vi "ONR Det Tube.vi"() -> ()   [LabVIEW 2018]
uses:
  <vilib>/Utility/miscctls.llb/LVPointTypeDef.ctl
  <vilib>/DAQmx/write.llb/DAQmx Write (Digital 1D Bool 1Chan 1Samp).vi
  <vilib>/Analysis/baseanly.llb/Mean (DBL).vi
  <vilib>/DAQmx/read.llb/DAQmx Read (Analog 1D Wfm NChan 1Samp).vi
  <vilib>/DAQmx/create/channels.llb/DAQmx Create Channel (DO-Digital Output).vi
  <vilib>/DAQmx/miscellaneous.llb/DAQmx Fill In Error Info.vi
  <vilib>/Utility/file.llb/Write Delimited Spreadsheet (string).vi
  <vilib>/Analysis/NI_AALBase.lvlib
panel:
  in  "Stop sensors":bool
  in  "Stop all":bool
  out "log_manifold_vent_end":timestamp
  out "log_manifold_vent_start":timestamp
  out "log_end_time":timestamp
  out "log_start_time":timestamp
  in  "Sensor sample period (ms)":i32=100
  in  "Vacuum Cutoff":dbl[unit]=3447.37894475789 caption="Nominal" format="%.2f"
  out "vac err":dbl caption="Error" format="%.3f %%"
  out "Diluent Cutoff (default)":dbl[unit] caption="Nominal" format="%.2f"
  out "Fuel Cutoff (default)":dbl[unit] caption="Nominal" format="%.2f"
  out "dil err":dbl caption="Error" format="%.3f %%"
  in  "Diluent underpressure":dbl[unit]=160.0 caption="Undershoot" format="%.2f"
  out "diode read status":string="Diode read N/A"
  out "Pressure Unsafe?":bool
  in  "Atmospheric Pressure":dbl[unit] format="%.2f"
  out "Tube Pressure":dbl[unit] format="%.2f"
  out "Tube Temp":dbl[unit]=294.2611111111111 format="%.2f"
  out "Ambient Temp":dbl[unit]=294.2611111111111 format="%.2f"
  in  "Plot Units":string(combo)="Pa"
  out "System Pressures":waveform(dbl)[](graph)
  in  "Spark":bool
  out "Test row":string[](array[string])
  in  "Diluent":string(combo)
  in  "Equivalence Ratio":string(combo)
  in  "Diluent Mole Fraction":string(combo)
  in  "Fuel":string(combo)
  in  "Initial Pressure":string(combo)
  in  "Oxidizer":string(combo)
  out "Test CSV":string[][](array[string])
  out "Test CSV Header":string[](array[string])
  out "indices":T1
  in  "Run Test":bool
  in  "Test condition CSV":path=path "C:/DAQ/test matrix.csv" caption="Test Conditions"
  out "tube ready?":bool
  out "Test Status":string="No tests loaded"
  out "log_vac_press":dbl[](array[numeric])
  out "log_vac_time":timestamp[](array[timestamp])
  out "log_vac_temp":dbl[](array[numeric])
  out "valve\nrefs":refnum<vi>[](array[refnum])
  out "log_dil_press":dbl[](array[numeric])
  out "log_dil_time":timestamp[](array[timestamp])
  out "log_dil_temp":dbl[](array[numeric])
  out "is diluted?":bool
  out "Vacuum Cutoff (actual)":dbl[unit] caption="Measured" format="%.2f"
  out "f_a_st":dbl caption="F/Ast" format="%.6f"
  out "Oxidizer Cutoff (default)":dbl[unit] caption="Nominal" format="%.2f"
  out "ox err":dbl caption="Error" format="%.3f %%"
  out "Diluent Cutoff (actual)":dbl[unit] caption="Measured" format="%.2f"
  out "Oxidizer Cutoff (actual)":dbl[unit] caption="Measured" format="%.2f"
  out "phi actual":dbl caption="Equivalence" format="%_6g"
  out "dil_mf_measured":dbl caption="Dilution" format="%_6g"
  out "log_ox_press":dbl[](array[numeric])
  out "log_ox_time":timestamp[](array[timestamp])
  out "log_ox_temp":dbl[](array[numeric])
  out "Manifold Temp":dbl[unit]=294.2611111111111 format="%.2f"
  out "Diluent Cutoff (adjusted)":dbl[unit] caption="Adjusted" format="%.2f"
  out "Fuel Cutoff (actual)":dbl[unit] caption="Measured" format="%.2f"
  out "log_fuel_press":dbl[](array[numeric])
  out "log_fuel_time":timestamp[](array[timestamp])
  out "log_fuel_temp":dbl[](array[numeric])
  in  "Pressure measure time":dbl[unit]=30.0
  out "Fuel Cutoff (adjusted)":dbl[unit] caption="Adjusted" format="%.2f"
  out "Manifold Pressure":dbl[unit] format="%.2f"
  out "fuel err":dbl caption="Error" format="%.3f %%"
  in  "Fuel underpressure":dbl[unit]=180.0 caption="Undershoot" format="%.2f"
  in  "Mix Fan":bool
  in  "Valve Tube Inlet":bool caption="Tube Inlet"
  in  "Valve Mix Inlet":bool caption="Mix Inlet"
  in  "Valve Mix Outlet":bool caption="Mix Outlet"
  in  "Valve Tube Outlet":bool=TRUE caption="Tube Outlet"
  in  "Valve Oxidizer":bool caption="Oxidizer"
  in  "Valve Fuel":bool caption="Fuel"
  in  "Valve Diluent":bool caption="Diluent"
  in  "Valve Purge":bool caption="Purge"
  in  "Valve Vacuum":bool caption="Vacuum"
  in  "Set Mode":bool=TRUE
  out "Remaining":dbl format="%<%M:%S>t"
  in  "Stop":bool
  in  "Mix Time":dbl[unit]=180.0 format="%#_13g"
  in  "Mix Section Purge":dbl[unit]=30.0 format="%#_13g"
  in  "Tube Purge":dbl[unit]=360.0 format="%#_13g"
  in  "Tube State":T2(ring)
  # "Timing"
  # "Vacuum"
  # "Diluent"
  # "Oxidizer"
  # "Fuel"
types:
  T1 = cluster{"fuel":i32, "oxidizer":i32, "diluent":i32, "diluent_mol_frac":i32, "equivalence":i32, "init_pressure":i32, "p_f":i32, "p_ox":i32, "p_dil":i32}
  T2 = enum16{"Tube Vent", "Mix Section Purge", "Tube Purge", "Tube Vacuum", "Diluent Fill", "Oxidizer Fill", "Fuel Fill", "Fill Hold", "Mixing", "Tube Closed", "Ignition", "Manifold Vent"}
  T3 = enum8{"Enabled", "Disabled", "Disabled and Grayed Out"}
  T4 = typedef "LVPointTypeDef.ctl" = cluster{"Horizontal":i16, "Vertical":i16}
  T5 = typedef "LVRangeTypeDef.ctl" = cluster{"Minimum":dbl, "Maximum":dbl, "Increment":dbl, "Minor Increment":dbl, "Start":dbl}
  T6 = enum16{"open", "open or create", "create or replace", "create", "open (read-only)"}
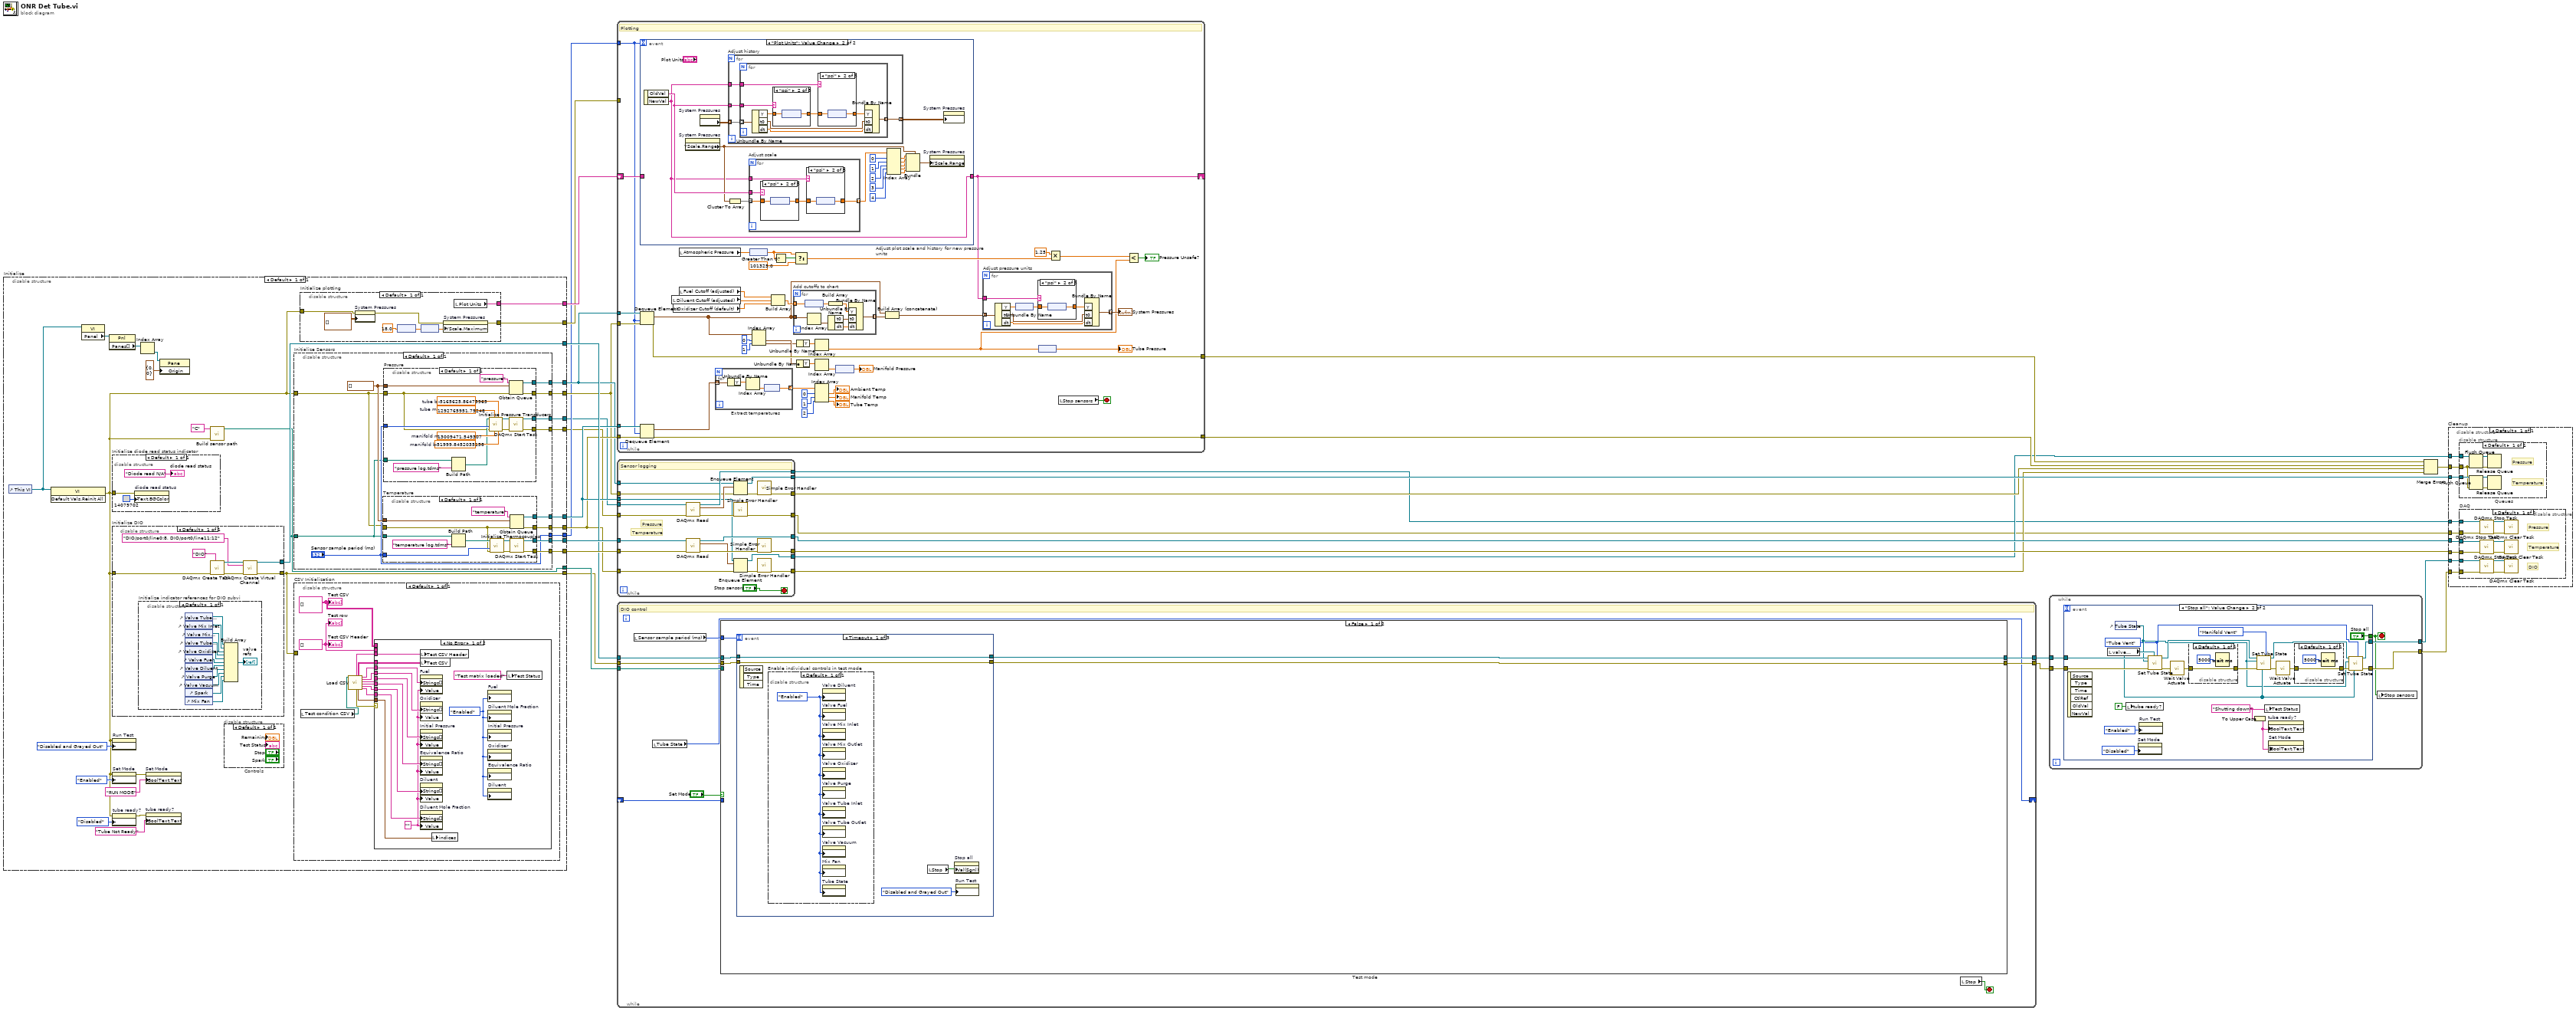
[diagram p0: block diagram]
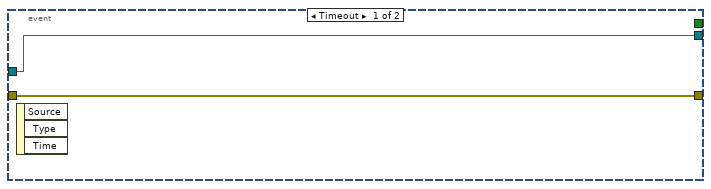
[diagram p2: hidden frame]
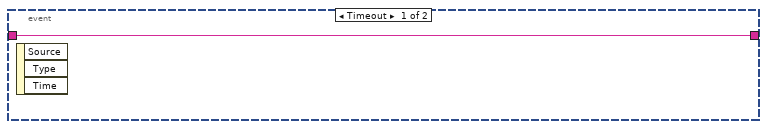
[diagram p4: hidden frame]
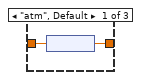
[diagram p5: hidden frame]
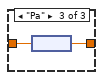
[diagram p6: hidden frame]
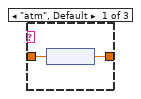
[diagram p7: hidden frame]
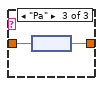
[diagram p8: hidden frame]
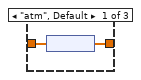
[diagram p9: hidden frame]
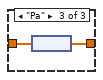
[diagram p10: hidden frame]
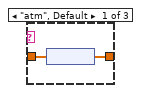
[diagram p11: hidden frame]
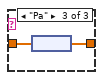
[diagram p12: hidden frame]
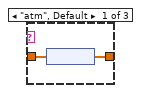
[diagram p13: hidden frame]
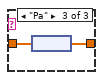
[diagram p14: hidden frame]
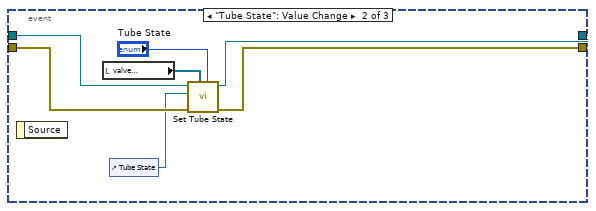
[diagram p15: hidden frame]
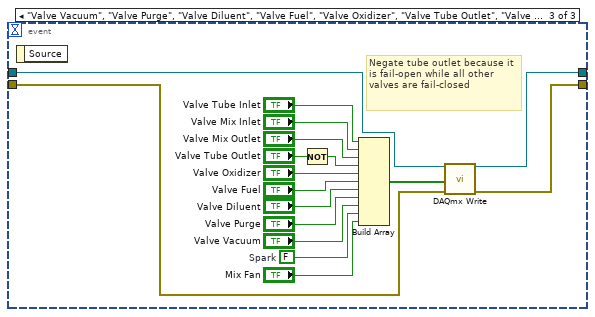
[diagram p16: hidden frame]
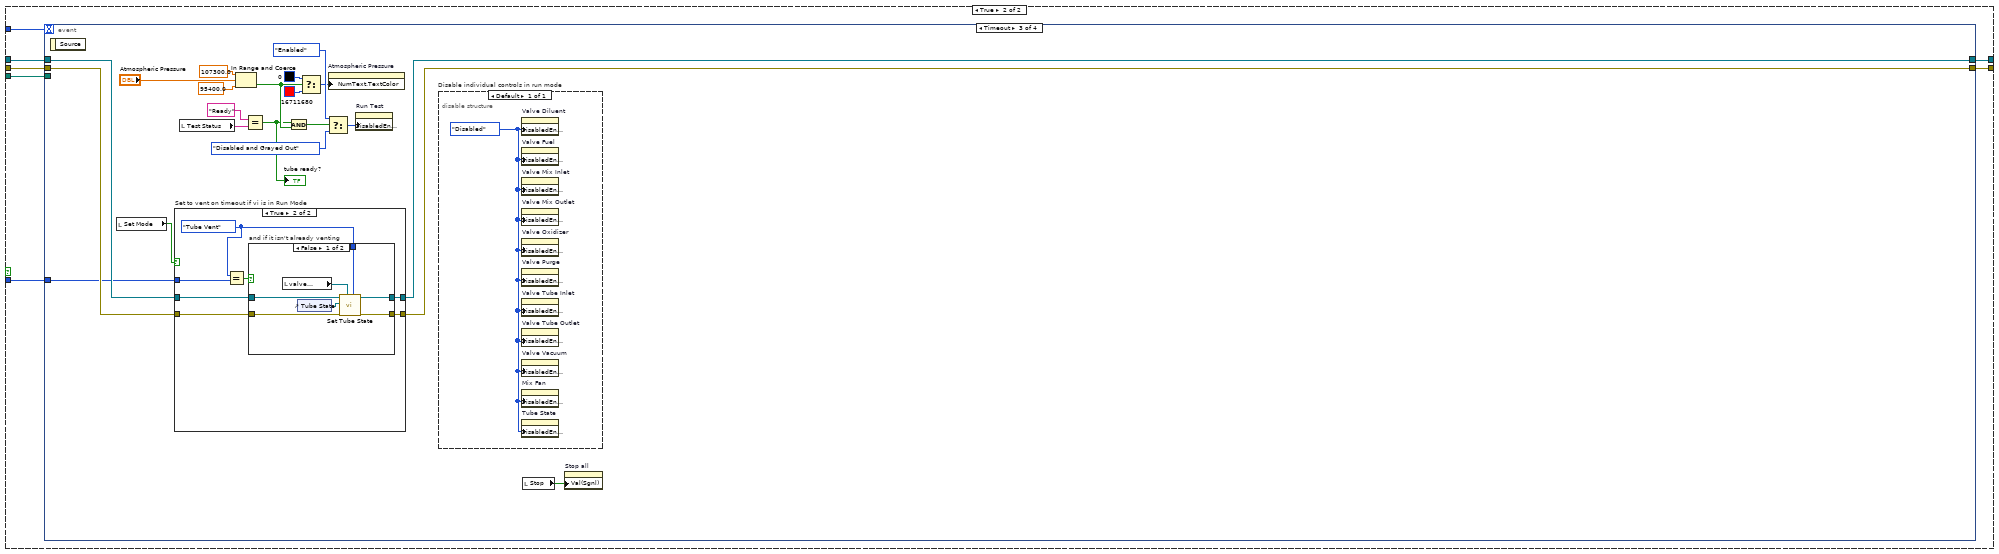
[diagram p17: hidden frame]
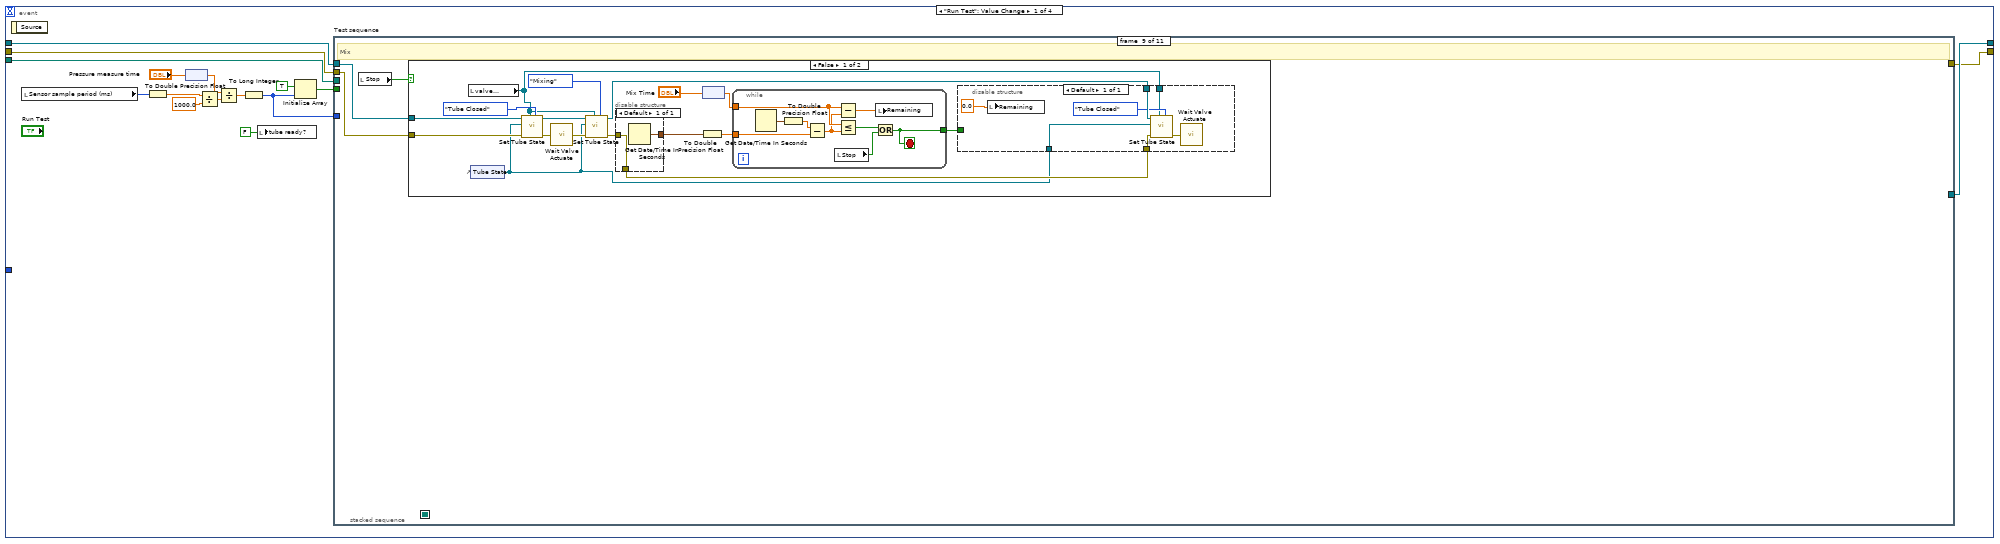
[diagram p18: hidden frame]
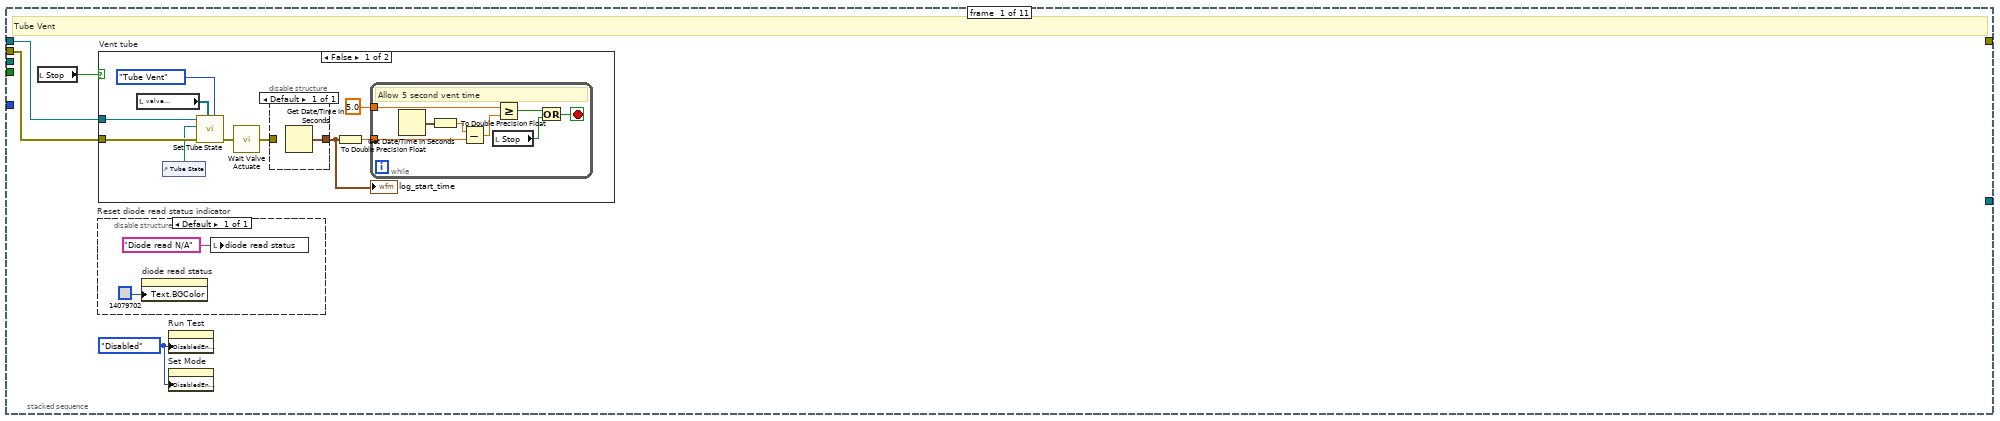
[diagram p19: hidden frame]
diagram:
  n1 = disable-structure "Initialize" shown="Default" {
    disable-tunnel: [w56] -> w28
    disable-tunnel: [w55] -> w26
    disable-tunnel: [w54] -> w22
    disable-tunnel: [w53] -> w21
    disable-tunnel: [w52] -> w20
    disable-tunnel: [w51] -> w16
    disable-tunnel: [w50] -> w15
    disable-tunnel: [w48] -> w14
    disable-tunnel: [w47] -> w13
    disable-tunnel: [w46] -> w12
    disable-tunnel: [w45] -> w11
    disable-tunnel: [w44] -> w10
    disable-tunnel: [w43] -> w9
    disable-tunnel: [w42] -> w8
    frame Enabled {
      n2 = control-ref of="This VI"() -> (w37:refnum<vi>)
      n3 = invoke class="VI" method="Default Vals.Reinit All"(reference=w37) -> (error out=w32:errorcluster)  [unwired: 2 in, 2 out]
      n4 = property class="VI"(reference=w37) -> ("Panel"=w38:refnum<vi>)  [unwired: 1 in, 2 out]
      n5 = property class="Pnl"(reference=w38) -> ("Panes[]"=w39:refnum<vi>[])  [unwired: 1 in, 2 out]
      n6 = disable-structure "Initialize diode read status indicator" shown="Default" {
        disable-tunnel: w32 -> [w152]
        frame Enabled {
          n7 = property on="diode read status" class="Str"(error in=w152, "Text.BGColor"=u32 14079702 ("Text.Colors:BG Color")) -> ()  [unwired: 1 in, 2 out]
          "diode read status" <- "Diode read N/A" ("diode read status")
        }
      }
      n8 = disable-structure "Initialize DIO" shown="Default" {
        disable-tunnel: [w87] -> w54
        disable-tunnel: [w84] -> w42
        disable-tunnel: w32 -> [w83]
        frame Enabled {
          n9 = disable-structure "Initialize indicator references for DIO subvi" shown="Default" {
            frame Enabled {
              n10 = control-ref of="Valve Tube Inlet"() -> (w101:refnum<vi>)
              n11 = control-ref of="Valve Mix Inlet"() -> (w100:refnum<vi>)
              n12 = control-ref of="Valve Mix Outlet"() -> (w99:refnum<vi>)
              n13 = control-ref of="Valve Tube Outlet"() -> (w98:refnum<vi>)
              n14 = control-ref of="Valve Oxidizer"() -> (w94:refnum<vi>)
              n15 = control-ref of="Valve Fuel"() -> (w93:refnum<vi>)
              n16 = control-ref of="Valve Diluent"() -> (w92:refnum<vi>)
              n17 = control-ref of="Valve Purge"() -> (w91:refnum<vi>)
              n18 = control-ref of="Valve Vacuum"() -> (w90:refnum<vi>)
              n19 = control-ref of="Spark"() -> (w95:refnum<vi>)
              n20 = control-ref of="Mix Fan"() -> (w96:refnum<vi>)
              n21 = Build Array(w101, w100, w99, w98, w94, w93, w92, w91, w90, w95, w96) -> (→"valve\nrefs":refnum<vi>[])
            }
          }
          n22 = call <vilib>:"DAQmx Create Task.vi"("new task name"="DIO", "error in"=w83) -> ("task out"=w88:refnum<k21>, "error out"=w86:errorcluster)  [unwired: 12 in]
          n23 = call-poly <vilib>:"DAQmx Create Virtual Channel.vi"("task in"=w88, "lines"=tag "DIO/port0/line0:8, DIO/port0/line11:12", "error in"=w86) -> ("task out"=w87:refnum<k21>, "error out"=w84:errorcluster)  [unwired: 11 in]
        }
      }
      n24 = property on="Run Test" class="Bool"(error in=w32, "DisabledEnum"=T3."Disabled and Grayed Out" ("Disabled")) -> ()  [unwired: 1 in, 2 out]
      n25 = property on="Set Mode" class="Bool (strict)"(error in=w32, "DisabledEnum"=T3."Enabled" ("Disabled")) -> (error out=w35:errorcluster)  [unwired: 1 in, 1 out]
      n26 = property on="tube ready?" class="Bool"(error in=w32, "DisabledEnum"=T3."Disabled" ("Disabled")) -> (error out=w31:errorcluster)  [unwired: 1 in, 1 out]
      n27 = Index Array(array=w39) -> (element=w40:refnum<vi>)  [unwired: 1 in]
      n28 = property on="Set Mode" class="Bool (strict)"(error in=w35, "BoolText.Text"="RUN MODE" ("Boolean Text.Text")) -> ()  [unwired: 1 in, 2 out]
      n29 = property on="tube ready?" class="Bool"(error in=w31, "BoolText.Text"="Tube Not Ready" ("Boolean Text.Text")) -> ()  [unwired: 1 in, 2 out]
      n30 = property class="Pane"(reference=w40, "Origin"=T4 {"Horizontal"=0, "Vertical"=0}) -> ()  [unwired: 1 in, 2 out]
      n31 = call "Build sensor path.vi"("Drive"="C", "error in"=w32) -> ("Current test directory"=w43:path)  [unwired: 7 in, 1 out]
      n32 = disable-structure "Controls" shown="Default" {
        frame Enabled {
        }
      }
      n33 = disable-structure "Initialize Sensors" shown="Default" {
        disable-tunnel: [w121] -> w56
        disable-tunnel: [w120] -> w55
        disable-tunnel: [w119] -> w51
        disable-tunnel: [w118] -> w50
        disable-tunnel: [w116] -> w48
        disable-tunnel: [w115] -> w47
        disable-tunnel: ["Sensor sample period (ms)"] -> w46
        disable-tunnel: [w113] -> w45
        disable-tunnel: [w112] -> w44
        disable-tunnel: w43 -> [w111]
        disable-tunnel: w32 -> [w110]
        frame Enabled {
          w117 = waveform(dbl)[] [] ("data")
          n34 = disable-structure "Temperature" shown="Default" {
            disable-tunnel: [w151] -> w121
            disable-tunnel: [w150] -> w120
            disable-tunnel: w111 -> [w146]
            disable-tunnel: [w143] -> w119
            disable-tunnel: [w142] -> w118
            disable-tunnel: "Sensor sample period (ms)" -> [w141]
            disable-tunnel: w117 -> [w140]
            disable-tunnel: w110 -> [w139]
            frame Enabled {
              n35 = Build Path(base path=w146, name or relative path="temperature log.tdms") -> (appended path=w145:path)
              n36 = call "Initialize Thermocouples.vi"("error in"=w139, "Sensor sample period (ms)"=w141, "file path"=w145) -> ("Error Out"=w149:errorcluster, "task out"=w148:refnum<k21>)  [unwired: 7 in]
              n37 = Obtain Queue(name (unnamed)="temperature", element data type=w140, error in (no error)=w139) -> (queue out=w143:refnum<queue>, error out=w142:errorcluster)  [unwired: 2 in, 1 out]
              n38 = call <vilib>:"DAQmx Start Task.vi"("task/channels in"=w148, "error in"=w149) -> ("task out"=w150:refnum<k21>, "error out"=w151:errorcluster)  [unwired: 12 in]
            }
          }
          n39 = disable-structure "Pressure" shown="Default" {
            disable-tunnel: w117 -> [w138]
            disable-tunnel: [w137] -> w116
            disable-tunnel: [w136] -> w115
            disable-tunnel: "Sensor sample period (ms)" -> [w134]
            disable-tunnel: [w127] -> w113
            disable-tunnel: [w126] -> w112
            disable-tunnel: w111 -> [w124]
            disable-tunnel: w110 -> [w122]
            frame Enabled {
              w132 = 13009471.549307  # manifold m
              w131 = -5165625.86475965  # tube b
              w130 = 1292765951.79248  # tube m
              w133 = -51999.8452035158  # manifold b
              n40 = Build Path(base path=w124, name or relative path="pressure log.tdms") -> (appended path=w123:path)
              n41 = call "Initialize Pressure Transducers.vi"("manifold b"=w133, "tube b"=w131, "manifold m"=w132, "tube m"=w130, "error in"=w122, "Sensor sample period (ms)"=w134, "file path"=w123) -> ("Error Out"=w128:errorcluster, "task out"=w129:refnum<k21>)  [unwired: 3 in]
              n42 = Obtain Queue(name (unnamed)="pressure", element data type=w138, error in (no error)=w122) -> (queue out=w137:refnum<queue>, error out=w136:errorcluster)  [unwired: 2 in, 1 out]
              n43 = call <vilib>:"DAQmx Start Task.vi"("task/channels in"=w129, "error in"=w128) -> ("task out"=w127:refnum<k21>, "error out"=w126:errorcluster)  [unwired: 12 in]
            }
          }
        }
      }
      n44 = disable-structure "CSV Initialization" shown="Default" {
        disable-tunnel: w42 -> [_]
        frame Enabled {
          w58 = string[][] []
          w59 = string[] []
          n45 = local read "Test condition CSV"() -> (w60:path)
          n46 = call "Load CSV.vi"("CSV Path"=w60) -> ("Header"=w70:string[], "error out"=w69:errorcluster, "CSV Array"=w68:string[][], "indices"=w67:T1, "Fuel"=w64:string[], "Oxidizer"=w65:string[], "Initial Pressure"=w66:string[], "Equivalence Ratio"=w63:string[], "Diluent"=w62:string[], "Diluent Mole Fraction"=w61:string[])  [unwired: 9 in]
          n47 = case shown="No Error" w69 {
            tunnel: w61 -> [w82 _]
            tunnel: w62 -> [w81 _]
            tunnel: w63 -> [w80 _]
            tunnel: w64 -> [w79 _]
            tunnel: w65 -> [w78 _]
            tunnel: w66 -> [w77 _]
            tunnel: w67 -> [w71 _]
            tunnel: w68 -> [w72 _]
            tunnel: w70 -> [w73 _]
            tunnel: w59 -> [_ _]
            tunnel: w58 -> [_ _]
            frame No Error {
              w74 = T3."Enabled" ("Disabled")
              w76 = "" ("Value (Signaling)")
              n48 = local write "Test CSV Header"(w73) -> ()
              n49 = local write "Test CSV"(w72) -> ()
              n50 = property on="Fuel" class="CmbBox"("Strings[]"=w79, "Value"=w76) -> ()  [unwired: 2 in, 2 out]
              n51 = property on="Oxidizer" class="CmbBox"("Strings[]"=w78, "Value"=w76) -> ()  [unwired: 2 in, 2 out]
              n52 = property on="Initial Pressure" class="CmbBox"("Strings[]"=w77, "Value"=w76) -> ()  [unwired: 2 in, 2 out]
              n53 = property on="Equivalence Ratio" class="CmbBox"("Strings[]"=w80, "Value"=w76) -> ()  [unwired: 2 in, 2 out]
              n54 = property on="Diluent" class="CmbBox"("Strings[]"=w81, "Value"=w76) -> ()  [unwired: 2 in, 2 out]
              n55 = property on="Diluent Mole Fraction" class="CmbBox"("Strings[]"=w82, "Value"=w76) -> ()  [unwired: 2 in, 2 out]
              n56 = local write "indices"(w71) -> ()
              n57 = property on="Fuel" class="CmbBox"("DisabledEnum"=w74) -> ()  [unwired: 2 in, 2 out]
              n58 = property on="Diluent Mole Fraction" class="CmbBox"("DisabledEnum"=w74) -> ()  [unwired: 2 in, 2 out]
              n59 = property on="Initial Pressure" class="CmbBox"("DisabledEnum"=w74) -> ()  [unwired: 2 in, 2 out]
              n60 = property on="Oxidizer" class="CmbBox"("DisabledEnum"=w74) -> ()  [unwired: 2 in, 2 out]
              n61 = property on="Equivalence Ratio" class="CmbBox"("DisabledEnum"=w74) -> ()  [unwired: 2 in, 2 out]
              n62 = property on="Diluent" class="CmbBox"("DisabledEnum"=w74) -> ()  [unwired: 2 in, 2 out]
              n63 = local write "Test Status"("Test matrix loaded" ("Test Status")) -> ()
            }
            frame Error {
            }
          }
          "Test CSV" <- w58
          "Test CSV Header" <- w59
          "Test row" <- w59
        }
      }
      n64 = disable-structure "Initialize plotting" shown="Default" {
        disable-tunnel: [w109] -> w53
        disable-tunnel: [w105] -> w52
        disable-tunnel: w32 -> [w102]
        frame Enabled {
          n65 = property on="System Pressures" class="WFChart (strict)"(error in=w102, "History Data"=waveform(dbl)[][] []) -> (error out=w103:errorcluster)  [unwired: 1 in, 1 out]
          n66 = node(18.0 ("Y Scale.Range:Maximum")) -> (w107:dbl[unit])
          n67 = node(w107) -> (w106:dbl)
          n68 = property on="System Pressures" class="WFChart (strict)"(error in=w103, "YScale.Maximum"=w106) -> (error out=w105:errorcluster)  [unwired: 1 in, 1 out]
          n69 = local read "Plot Units"() -> (w109:string)
        }
      }
    }
  }
  n70 = while {
    tunnel: w14 -> [w198]
    tunnel: [w196] -> w24
    shift-right: [w155] -> _
    shift-left: w21 -> [w193]
    tunnel: w20 -> [_]
    tunnel: [w165] -> w17
    tunnel: w16 -> [w168]
    tunnel: w13 -> [w167]
    tunnel: w15 -> [w166]
    tunnel: w12 -> [w156]
    stop <- w197 stop-if-true
    # "Plotting"
    n71 = event "Adjust plot scale and history for new pressure units" shown="[1] \"Plot Units\": Value Change" {
      selector: _ -> [_ _]
      dyn-events: _ -> [_ _]
      timeout: w156 -> [_ _]
      tunnel: w193 -> [w211 _]
      tunnel: [w211 w212] -> w155
      event Timeout {
        n72 = event-data() -> ()  [unwired: 1 in, 3 out]
      }
      event "Plot Units": Value Change {
        n73 = event-data() -> ("OldVal"=w227:string, "NewVal"=w212:string)  [unwired: 1 in]
        n74 = property on="System Pressures" class="WFChart (strict)"() -> ("YScale.Range"=w224:T5)  [unwired: 2 in, 2 out]
        n75 = property on="System Pressures" class="WFChart (strict)"() -> ("History Data"=w229:waveform(dbl)[][])  [unwired: 2 in, 2 out]
        n76 = for "Adjust history" {
          tunnel: w229 -> [w250] mode=indexing
          tunnel: [w249] -> w228 mode=indexing
          tunnel: w227 -> [w248]
          tunnel: w212 -> [w247]
          n77 = for {
            tunnel: w250 -> [w259] mode=indexing
            tunnel: [w256] -> w249 mode=indexing
            tunnel: w248 -> [w255]
            tunnel: w247 -> [w254]
            n78 = Unbundle By Name(w259) -> ("Y"=w252:dbl[], "t0"=w258:timestamp, "dt"=w257:dbl)
            n79 = case shown="\"psi\"" w255 {
              tunnel: [w267 w269 w271] -> w253
              tunnel: w252 -> [w266 w268 w270]
              frame "atm", Default {
                n80 = node(w266) -> (w267:dbl[unit][])
              }
              frame "psi" {
                n81 = node(w268) -> (w269:dbl[unit][])
              }
              frame "Pa" {
                n82 = node(w270) -> (w271:dbl[unit][])
              }
            }
            n83 = case shown="\"psi\"" w254 {
              tunnel: w253 -> [w261 w263 w265]
              tunnel: [w260 w262 w264] -> w251
              frame "atm", Default {
                n84 = node(w261) -> (w260:dbl[])
              }
              frame "psi" {
                n85 = node(w263) -> (w262:dbl[])
              }
              frame "Pa" {
                n86 = node(w265) -> (w264:dbl[])
              }
            }
            n87 = Bundle By Name("Y"=w251, "t0"=w258, "dt"=w257) -> (w256:waveform(dbl))  [unwired: 1 in]
          }
        }
        n88 = Cluster To Array(cluster=w224) -> (array=w226:dbl[])
        n89 = for "Adjust scale" {
          tunnel: w212 -> [w233]
          tunnel: w227 -> [w232]
          tunnel: w226 -> [w231] mode=indexing
          tunnel: [w230] -> w222 mode=indexing
          n90 = case shown="\"psi\"" w232 {
            tunnel: [w242 w244 w246] -> w234
            tunnel: w231 -> [w241 w243 w245]
            frame "atm", Default {
              n91 = node(w241) -> (w242:dbl[unit])
            }
            frame "psi" {
              n92 = node(w243) -> (w244:dbl[unit])
            }
            frame "Pa" {
              n93 = node(w245) -> (w246:dbl[unit])
            }
          }
          n94 = case shown="\"psi\"" w233 {
            tunnel: w234 -> [w236 w238 w240]
            tunnel: [w235 w237 w239] -> w230
            frame "atm", Default {
              n95 = node(w236) -> (w235:dbl)
            }
            frame "psi" {
              n96 = node(w238) -> (w237:dbl)
            }
            frame "Pa" {
              n97 = node(w240) -> (w239:dbl)
            }
          }
        }
        n98 = Index Array(array=w222, index #1=0 ("index"), index #2=1 ("index"), index #3=2 ("index"), index #4=3 ("index"), index #5=4 ("index")) -> (element #1=w223:dbl, element #2=w221:dbl, element #3=w220:dbl, element #4=w219:dbl, element #5=w218:dbl)
        n99 = Bundle(cluster=w224, "Minimum"=w223, "Maximum"=w221, "Increment"=w220, "Minor Increment"=w219, "Start"=w218) -> (w225:T5)
        n100 = property on="System Pressures" class="WFChart (strict)"("YScale.Range"=w225) -> ()  [unwired: 2 in, 2 out]
        n101 = property on="System Pressures" class="WFChart (strict)"("History Data"=w228) -> ()  [unwired: 2 in, 2 out]
      }
    }
    n102 = Dequeue Element(queue=w198, timeout in ms (-1)=w156, error in (no error)=w167) -> (element=w187:waveform(dbl)[], error out=w196:errorcluster)  [unwired: 2 out]
    n103 = Dequeue Element(queue=w168, timeout in ms (-1)=w156, error in (no error)=w166) -> (element=w164:waveform(dbl)[], error out=w165:errorcluster)  [unwired: 2 out]
    n104 = local read "Diluent Cutoff (adjusted)"() -> (w190:dbl[unit])
    n105 = local read "Oxidizer Cutoff (default)"() -> (w191:dbl[unit])
    n106 = local read "Atmospheric Pressure"() -> (w174:dbl[unit])
    n107 = local read "Fuel Cutoff (adjusted)"() -> (w192:dbl[unit])
    n108 = for "Extract temperatures" {
      tunnel: w164 -> [w202] mode=indexing
      tunnel: [w199] -> w157 mode=indexing
      n109 = Unbundle By Name(w202) -> ("Y"=w201:dbl[])
      n110 = Index Array(array=w201) -> (element=w200:dbl)  [unwired: 1 in]
      n111 = node(w200) -> (w199:dbl[unit])
    }
    n112 = node(w174) -> (w173:dbl)
    n113 = Index Array(array=w187, index #1=0 ("index"), index #2=1 ("index")) -> (element #1=w184:waveform(dbl), element #2=w183:waveform(dbl))
    n114 = Build Array(w192, w190, w191) -> (w189:dbl[unit][])
    n115 = Greater Than 0?(x=w173) -> (x > 0?=w175:bool)
    n116 = for "Add cutoffs to chart" {
      tunnel: w187 -> [w209]
      tunnel: w189 -> [w204] mode=indexing
      tunnel: [w203] -> w188 mode=indexing
      n117 = node(w204) -> (w206:dbl)
      n118 = Index Array(array=w209) -> (element=w210:waveform(dbl))  [unwired: 1 in]
      n119 = Unbundle By Name(w210) -> ("t0"=w207:timestamp, "dt"=w208:dbl)
      n120 = Build Array(w206) -> (w205:dbl[])
      n121 = Bundle By Name("Y"=w205, "t0"=w207, "dt"=w208) -> (w203:waveform(dbl))  [unwired: 1 in]
    }
    n122 = Select(t=w173, s=w175, f=101325.0) -> (s? t:f=w171:dbl)
    n123 = Unbundle By Name(w183) -> ("Y"=w179:dbl[])
    n124 = Unbundle By Name(w184) -> ("Y"=w182:dbl[])
    n125 = Index Array(array=w179) -> (element=w170:dbl)  [unwired: 1 in]
    n126 = Index Array(array=w182) -> (element=w181:dbl)  [unwired: 1 in]
    n127 = Index Array(array=w157, index #1=0 ("index"), index #2=1 ("index"), index #3=2 ("index")) -> (element #1=→"Ambient Temp":dbl[unit], element #2=→"Manifold Temp":dbl[unit], element #3=→"Tube Temp":dbl[unit])
    n128 = node(w181) -> (→"Manifold Pressure":dbl[unit])
    n129 = Build Array (concatenate)(w187, w188) -> (w195:waveform(dbl)[])
    n130 = for "Adjust pressure units" {
      tunnel: w155 -> [w279]
      tunnel: w195 -> [w276] mode=indexing
      tunnel: [w272] -> w194 mode=indexing
      n131 = Unbundle By Name(w276) -> ("Y"=w275:dbl[], "t0"=w278:timestamp, "dt"=w277:dbl)
      n132 = node(w275) -> (w274:dbl[unit][])
      n133 = case shown="\"psi\"" w279 {
        tunnel: w274 -> [w280 w283 w284]
        tunnel: [w281 w282 w285] -> w273
        frame "atm", Default {
          n134 = node(w280) -> (w281:dbl[])
        }
        frame "psi" {
          n135 = node(w283) -> (w282:dbl[])
        }
        frame "Pa" {
          n136 = node(w284) -> (w285:dbl[])
        }
      }
      n137 = Bundle By Name("Y"=w273, "t0"=w278, "dt"=w277) -> (w272:waveform(dbl))  [unwired: 1 in]
    }
    "System Pressures" <- w194
    n138 = node(w170) -> (→"Tube Pressure":dbl[unit])
    n139 = Multiply(x=1.25, y=w171) -> (x*y=w177:dbl)
    n140 = local read "Stop sensors"() -> (w197:bool)
    n141 = Less?(x=w177, y=w170) -> (x < y?=→"Pressure Unsafe?":bool)
  }
  n142 = while {
    tunnel: w11 -> [w304]
    tunnel: [w301] -> w6
    tunnel: w10 -> [w303]
    tunnel: [w293] -> w5
    tunnel: w26 -> [w306]
    tunnel: [w305] -> w27
    tunnel: w28 -> [w308]
    tunnel: [w294] -> w29
    tunnel: w14 -> [w300]
    tunnel: [w298] -> w25
    tunnel: [w295] -> w18
    tunnel: w13 -> [w296]
    tunnel: w15 -> [w287]
    tunnel: w16 -> [w292]
    tunnel: [w290] -> w7
    tunnel: [w288] -> w19
    stop <- "Stop sensors" stop-if-true
    # "Pressure"
    # "Temperature"
    # "Sensor logging"
    n143 = call-poly <vilib>:"DAQmx Read.vi"("task/channels in"=w304, "error in"=w303) -> ("task out"=w301:refnum<k21>, "data"=w299:waveform(dbl)[], "error out"=w302:errorcluster)  [unwired: 11 in]
    n144 = call-poly <vilib>:"DAQmx Read.vi"("task/channels in"=w306, "error in"=w308) -> ("task out"=w305:refnum<k21>, "data"=w291:waveform(dbl)[], "error out"=w307:errorcluster)  [unwired: 11 in]
    n145 = Enqueue Element(queue=w300, element=w299, error in (no error)=w296) -> (queue out=w298:refnum<queue>, error out=w297:errorcluster)  [unwired: 1 in, 1 out]
    n146 = call <vilib>:"Simple Error Handler.vi"("error in (no error)"=w302) -> ("error out"=w293:errorcluster)  [unwired: 4 in, 4 out]
    n147 = Enqueue Element(queue=w292, element=w291, error in (no error)=w287) -> (queue out=w290:refnum<queue>, error out=w289:errorcluster)  [unwired: 1 in, 1 out]
    n148 = call <vilib>:"Simple Error Handler.vi"("error in (no error)"=w297) -> ("error out"=w295:errorcluster)  [unwired: 4 in, 4 out]
    n149 = call <vilib>:"Simple Error Handler.vi"("error in (no error)"=w307) -> ("error out"=w294:errorcluster)  [unwired: 4 in, 4 out]
    n150 = call <vilib>:"Simple Error Handler.vi"("error in (no error)"=w289) -> ("error out"=w288:errorcluster)  [unwired: 4 in, 4 out]
  }
  n151 = while {
    tunnel: w9 -> [w315]
    tunnel: w22 -> [w317]
    tunnel: [w318] -> w3
    tunnel: w8 -> [w316]
    tunnel: [w313] -> w4
    shift-right: [w310] -> _
    shift-left: _ -> [w309]
    stop <- w314 stop-if-true
    # "DIO control"
    n152 = local read "Sensor sample period (ms)"() -> (w311:i32)
    n153 = local read "Tube State"() -> (w310:T2)
    n154 = case "Test mode" shown="False" "Set Mode" {
      tunnel: [w319 w359] -> w318
      tunnel: w317 -> [w322 w358]
      tunnel: w316 -> [w321 w357]
      tunnel: w315 -> [_ w356]
      tunnel: [w320 w355] -> w313
      tunnel: w311 -> [w323 w354]
      tunnel: w309 -> [_ w353]
      frame False {
        n155 = event shown="[0] Timeout" {
          selector: _ -> [_ _ _]
          dyn-events: _ -> [_ _ _]
          timeout: w323 -> [_ _ _]
          tunnel: w322 -> [w327 w333 w338]
          tunnel: w321 -> [w326 w332 w339]
          tunnel: [w327 w331 w336] -> w319
          tunnel: [w326 w330 w337] -> w320
          event Timeout {
            n156 = event-data() -> ()  [unwired: 1 in, 3 out]
            n157 = disable-structure "Enable individual controls in test mode" shown="Default" {
              frame Enabled {
                w328 = T3."Enabled" ("Disabled")
                n158 = property on="Valve Diluent" class="Bool (strict)"("DisabledEnum"=w328) -> ()  [unwired: 2 in, 2 out]
                n159 = property on="Valve Fuel" class="Bool (strict)"("DisabledEnum"=w328) -> ()  [unwired: 2 in, 2 out]
                n160 = property on="Valve Mix Inlet" class="Bool (strict)"("DisabledEnum"=w328) -> ()  [unwired: 2 in, 2 out]
                n161 = property on="Valve Mix Outlet" class="Bool (strict)"("DisabledEnum"=w328) -> ()  [unwired: 2 in, 2 out]
                n162 = property on="Valve Oxidizer" class="Bool (strict)"("DisabledEnum"=w328) -> ()  [unwired: 2 in, 2 out]
                n163 = property on="Valve Purge" class="Bool (strict)"("DisabledEnum"=w328) -> ()  [unwired: 2 in, 2 out]
                n164 = property on="Valve Tube Inlet" class="Bool (strict)"("DisabledEnum"=w328) -> ()  [unwired: 2 in, 2 out]
                n165 = property on="Valve Tube Outlet" class="Bool (strict)"("DisabledEnum"=w328) -> ()  [unwired: 2 in, 2 out]
                n166 = property on="Valve Vacuum" class="Bool (strict)"("DisabledEnum"=w328) -> ()  [unwired: 2 in, 2 out]
                n167 = property on="Mix Fan" class="Bool (strict)"("DisabledEnum"=w328) -> ()  [unwired: 2 in, 2 out]
                n168 = property on="Tube State" class="Enum (strict)"("DisabledEnum"=w328) -> ()  [unwired: 2 in, 2 out]
              }
            }
            n169 = local read "Stop"() -> (w324:bool)
            n170 = property on="Stop all" class="Bool (strict)"("Val(Sgnl)"=w324) -> ()  [unwired: 2 in, 2 out]
            n171 = property on="Run Test" class="Bool"("DisabledEnum"=T3."Disabled and Grayed Out" ("Disabled")) -> ()  [unwired: 2 in, 2 out]
          }
          event "Tube State": Value Change {
            n172 = event-data() -> ()  [unwired: 1 in, 1 out]
            n173 = local read "valve\nrefs"() -> (w334:refnum<vi>[])
            n174 = control-ref of="Tube State"() -> (w329:refnum<vi>)
            n175 = call "Set Tube State.vi"("State"="Tube State", "valve refs"=w334, "error in"=w332, "tube state ref"=w329, "task in"=w333) -> ("error out"=w330:errorcluster, "task out"=w331:refnum<k21>)  [unwired: 3 in]
          }
          event "Valve Vacuum", "Valve Purge", "Valve Diluent", "Valve Fuel", "Valve Oxidizer", "Valve Tube Outlet", "Valve Mix Outlet", "Valve Mix Inlet", "Valve Tube Inlet", "Mix Fan": Value Change {
            w342 = FALSE  # Spark
            # "Negate tube outlet because it is fail-open while all other valves are fail-closed"
            n176 = event-data() -> ()  [unwired: 1 in, 1 out]
            n177 = Not(x="Valve Tube Outlet") -> (.not. x?=w348:bool)
            n178 = Build Array("Valve Tube Inlet", "Valve Mix Inlet", "Valve Mix Outlet", w348, "Valve Oxidizer", "Valve Fuel", "Valve Diluent", "Valve Purge", "Valve Vacuum", w342, "Mix Fan") -> (w340:bool[])
            n179 = call-poly <vilib>:"DAQmx Write.vi"("task/channels in"=w338, "data"=w340, "error in"=w339) -> ("task out"=w336:refnum<k21>, "error out"=w337:errorcluster)  [unwired: 10 in, 1 out]
          }
        }
      }
      frame True {
        n180 = event shown="[2] Timeout" {
          selector: _ -> [_ _ _ _]
          dyn-events: _ -> [_ _ _ _]
          timeout: w354 -> [_ _ _ _]
          tunnel: [w367 w1071 w1113 w1158] -> w359
          tunnel: [w366 w1070 w1112 w1159] -> w355
          tunnel: w358 -> [w365 w1071 w1115 w1158]
          tunnel: w357 -> [w364 w1070 w1114 w1159]
          tunnel: w356 -> [w363 _ _ _]
          tunnel: w353 -> [_ _ w1096 _]
          event "Run Test": Value Change {
            n181 = event-data() -> ()  [unwired: 1 in, 1 out]
            n182 = local read "Sensor sample period (ms)"() -> (w374:i32)
            n183 = To Double Precision Float(number=w374) -> (double precision float=w361:dbl)
            n184 = node("Pressure measure time") -> (w362:dbl)
            n185 = Divide(x=w361, y=1000.0 ("x")) -> (x/y=w375:dbl)
            n186 = Divide(x=w362, y=w375) -> (x/y=w372:dbl)
            n187 = To Long Integer(number=w372) -> (32bit integer=w369:i32)
            n188 = local write "tube ready?"(FALSE ("tube ready?")) -> ()
            n189 = Initialize Array(TRUE, w369) -> (w368:bool[])
            n190 = stacked-sequence "Test sequence" {
              seq-local: [_ _ _ _ _ _ _ _ _ w923 _] -> [_ _ _ _ _ _ _ _ _ _ w1006]
              tunnel: w364 -> [w378 w403 w426 w451 w478 w585 w677 w784 w885 w924 w1009]
              tunnel: w365 -> [w379 w402 w427 w452 w479 w586 w678 w785 w886 w925 w1010]
              tunnel: w369 -> [_ _ _ _ w476 w583 w675 w782 _ _ _]
              tunnel: w368 -> [_ _ _ _ w475 w582 w674 w781 _ _ _]
              tunnel: w363 -> [_ _ _ _ _ _ _ _ _ w926 _]
              tunnel: [_ _ _ _ _ _ _ _ _ _ w1008] -> w366
              tunnel: [_ _ _ _ _ _ _ _ _ _ w1007] -> w367
              frame #0 {
                w376 = T3."Disabled" ("Disabled")
                # "Tube Vent"
                n191 = local read "Stop"() -> (w377:bool)
                n192 = disable-structure "Reset diode read status indicator" shown="Default" {
                  frame Enabled {
                    n193 = property on="diode read status" class="Str"("Text.BGColor"=u32 14079702 ("Text.Colors:BG Color")) -> ()  [unwired: 2 in, 2 out]
                    n194 = local write "diode read status"("Diode read N/A" ("diode read status")) -> ()
                  }
                }
                n195 = case "Vent tube" shown="False" w377 {
                  tunnel: w379 -> [w388 _]
                  tunnel: w378 -> [w387 _]
                  frame False {
                    n196 = local read "valve\nrefs"() -> (w385:refnum<vi>[])
                    n197 = control-ref of="Tube State"() -> (w382:refnum<vi>)
                    n198 = call "Set Tube State.vi"("State"=T2."Tube Vent", "valve refs"=w385, "error in"=w387, "tube state ref"=w382, "task in"=w388) -> ("error out"=w386:errorcluster)  [unwired: 3 in, 1 out]
                    n199 = call "Wait Valve Actuate.vi"("error in"=w386) -> ("error out"=w389:errorcluster)
                    n200 = disable-structure shown="Default" {
                      disable-tunnel: [w392] -> w391
                      disable-tunnel: w389 -> [_]
                      frame Enabled {
                        n201 = Get Date/Time In Seconds() -> (seconds since 1Jan1904=w392:timestamp)
                      }
                    }
                    "log_start_time" <- w391
                    n202 = To Double Precision Float(number=w391) -> (double precision float=w383:dbl)
                    n203 = while {
                      tunnel: w383 -> [w399]
                      tunnel: 5.0 -> [w397]
                      stop <- w395 stop-if-true
                      # "Allow 5 second vent time"
                      n204 = Get Date/Time In Seconds() -> (seconds since 1Jan1904=w400:timestamp)
                      n205 = To Double Precision Float(number=w400) -> (double precision float=w393:dbl)
                      n206 = Subtract(x=w393, y=w399) -> (x-y=w398:dbl)
                      n207 = local read "Stop"() -> (w394:bool)
                      n208 = Greater Or Equal?(x=w397, y=w398) -> (x >= y?=w396:bool)
                      n209 = Or(x=w396, y=w394) -> (x .or. y?=w395:bool)
                    }
                  }
                  frame True {
                  }
                }
                n210 = property on="Run Test" class="Bool"("DisabledEnum"=w376) -> ()  [unwired: 2 in, 2 out]
                n211 = property on="Set Mode" class="Bool (strict)"("DisabledEnum"=w376) -> ()  [unwired: 2 in, 2 out]
              }
              frame #1 {
                # "Manifold Vent"
                n212 = local read "Stop"() -> (w401:bool)
                n213 = case shown="False" w401 {
                  tunnel: w403 -> [w408 _]
                  tunnel: w402 -> [w409 _]
                  frame False {
                    n214 = local read "valve\nrefs"() -> (w411:refnum<vi>[])
                    n215 = control-ref of="Tube State"() -> (w404:refnum<vi>)
                    n216 = call "Set Tube State.vi"("State"=T2."Manifold Vent", "valve refs"=w411, "error in"=w408, "tube state ref"=w404, "task in"=w409) -> ("error out"=w407:errorcluster)  [unwired: 3 in, 1 out]
                    n217 = call "Wait Valve Actuate.vi"("error in"=w407) -> ("error out"=w412:errorcluster)
                    n218 = disable-structure shown="Default" {
                      disable-tunnel: [w415] -> w414
                      disable-tunnel: w412 -> [_]
                      frame Enabled {
                        n219 = Get Date/Time In Seconds() -> (seconds since 1Jan1904=w415:timestamp)
                      }
                    }
                    "log_manifold_vent_start" <- w414
                    n220 = To Double Precision Float(number=w414) -> (double precision float=w406:dbl)
                    n221 = while {
                      tunnel: w406 -> [w423]
                      tunnel: 5.0 -> [w421]
                      tunnel: [w416] -> w405
                      stop <- w419 stop-if-true
                      # "Allow 5 second vent time"
                      n222 = Get Date/Time In Seconds() -> (seconds since 1Jan1904=w424:timestamp)
                      n223 = To Double Precision Float(number=w424) -> (double precision float=w417:dbl)
                      n224 = Subtract(x=w417, y=w423) -> (x-y=w422:dbl)
                      n225 = local read "Stop"() -> (w418:bool)
                      n226 = Less Or Equal?(x=w421, y=w422) -> (x <= y?=w420:bool)
                      n227 = Or(x=w420, y=w418) -> (x .or. y?=w419:bool)
                      n228 = Get Date/Time In Seconds() -> (seconds since 1Jan1904=w416:timestamp)
                    }
                    "log_manifold_vent_end" <- w405
                  }
                  frame True {
                  }
                }
              }
              frame #2 {
                # "Tube Purge"
                n229 = local read "Stop"() -> (w425:bool)
                n230 = case shown="False" w425 {
                  tunnel: w427 -> [w432 _]
                  tunnel: w426 -> [w434 _]
                  frame False {
                    n231 = local read "valve\nrefs"() -> (w431:refnum<vi>[])
                    n232 = control-ref of="Tube State"() -> (w428:refnum<vi>)
                    n233 = call "Set Tube State.vi"("State"=T2."Tube Purge", "valve refs"=w431, "error in"=w434, "tube state ref"=w428, "task in"=w432) -> ("error out"=w433:errorcluster)  [unwired: 3 in, 1 out]
                    n234 = disable-structure shown="Default" {
                      disable-tunnel: [w440] -> w438
                      disable-tunnel: w433 -> [_]
                      frame Enabled {
                        n235 = Get Date/Time In Seconds() -> (seconds since 1Jan1904=w440:timestamp)
                      }
                    }
                    n236 = To Double Precision Float(number=w438) -> (double precision float=w429:dbl)
                    n237 = node("Tube Purge") -> (w435:dbl)
                    n238 = while {
                      tunnel: w429 -> [w448]
                      tunnel: [w445] -> w437
                      tunnel: w435 -> [w444]
                      stop <- w445 stop-if-true
                      n239 = Get Date/Time In Seconds() -> (seconds since 1Jan1904=w449:timestamp)
                      n240 = To Double Precision Float(number=w449) -> (double precision float=w441:dbl)
                      n241 = Subtract(x=w441, y=w448) -> (x-y=w443:dbl)
                      n242 = local read "Stop"() -> (w447:bool)
                      n243 = Subtract(x=w444, y=w443) -> (x-y=w442:dbl)
                      n244 = Less Or Equal?(x=w444, y=w443) -> (x <= y?=w446:bool)
                      n245 = Or(x=w446, y=w447) -> (x .or. y?=w445:bool)
                      n246 = local write "Remaining"(w442) -> ()
                    }
                    n247 = disable-structure shown="Default" {
                      disable-tunnel: w437 -> [_]
                      frame Enabled {
                        n248 = local write "Remaining"(0.0 ("Remaining")) -> ()
                      }
                    }
                  }
                  frame True {
                  }
                }
              }
              frame #3 {
                # "Mix Section Purge"
                n249 = local read "Stop"() -> (w450:bool)
                n250 = case shown="False" w450 {
                  tunnel: w452 -> [w457 _]
                  tunnel: w451 -> [w456 _]
                  frame False {
                    n251 = control-ref of="Tube State"() -> (w453:refnum<vi>)
                    n252 = local read "valve\nrefs"() -> (w458:refnum<vi>[])
                    n253 = call "Set Tube State.vi"("State"=T2."Mix Section Purge", "valve refs"=w458, "error in"=w456, "tube state ref"=w453, "task in"=w457) -> ("error out"=w455:errorcluster)  [unwired: 3 in, 1 out]
                    n254 = disable-structure shown="Default" {
                      disable-tunnel: [w465] -> w463
                      disable-tunnel: w455 -> [_]
                      frame Enabled {
                        n255 = Get Date/Time In Seconds() -> (seconds since 1Jan1904=w465:timestamp)
                      }
                    }
                    n256 = To Double Precision Float(number=w463) -> (double precision float=w454:dbl)
                    n257 = node("Mix Section Purge") -> (w462:dbl)
                    n258 = while {
                      tunnel: w454 -> [w473]
                      tunnel: w462 -> [w469]
                      tunnel: [w470] -> w460
                      stop <- w470 stop-if-true
                      n259 = Get Date/Time In Seconds() -> (seconds since 1Jan1904=w474:timestamp)
                      n260 = To Double Precision Float(number=w474) -> (double precision float=w466:dbl)
                      n261 = Subtract(x=w466, y=w473) -> (x-y=w468:dbl)
                      n262 = local read "Stop"() -> (w471:bool)
                      n263 = Subtract(x=w469, y=w468) -> (x-y=w467:dbl)
                      n264 = Less Or Equal?(x=w469, y=w468) -> (x <= y?=w472:bool)
                      n265 = Or(x=w472, y=w471) -> (x .or. y?=w470:bool)
                      n266 = local write "Remaining"(w467) -> ()
                    }
                    n267 = disable-structure shown="Default" {
                      disable-tunnel: w460 -> [_]
                      frame Enabled {
                        n268 = local write "Remaining"(0.0 ("Remaining")) -> ()
                      }
                    }
                  }
                  frame True {
                  }
                }
              }
              frame #4 {
                # "Tube Vacuum"
                n269 = local read "Stop"() -> (w477:bool)
                n270 = case shown="False" w477 {
                  tunnel: w479 -> [w489 _]
                  tunnel: w478 -> [w488 _]
                  tunnel: w476 -> [w485 _]
                  tunnel: w475 -> [w483 _]
                  frame False {
                    n271 = To Double Precision Float(number=w485) -> (double precision float=w487:dbl)
                    n272 = local read "Sensor sample period (ms)"() -> (w480:i32)
                    n273 = Decrement(x=w485) -> (x-1=w486:i32)
                    n274 = Reciprocal(x=w487) -> (1/x=w484:dbl)
                    n275 = To Unsigned Long Integer(number=w480) -> (unsigned 32bit integer=w481:u32)
                    n276 = while {
                      tunnel: w486 -> [w562]
                      shift-right: [w560] -> _
                      shift-left: w483 -> [w561]
                      tunnel: w484 -> [w559]
                      tunnel: w489 -> [w543]
                      tunnel: w488 -> [w542]
                      tunnel: [w541] -> w482
                      shift-right: [w536] -> _
                      shift-left: _ -> [w535]
                      tunnel: w481 -> [w534]
                      stop <- w541 stop-if-true
                      # "Tube vacuum"
                      n277 = local read "Manifold Pressure"() -> (w552:dbl[unit])
                      n278 = local read "Manifold Pressure"() -> (w544:dbl[unit])
                      n279 = local read "Vacuum Cutoff"() -> (w539:dbl[unit])
                      n280 = local read "Vacuum Cutoff"() -> (w540:dbl[unit])
                      n281 = Array Subset(array=w561, index=1, length=w562) -> (w548:bool[])
                      n282 = Subtract(x=w552, y=w539) -> (x-y=w555:dbl[unit])
                      n283 = call "Vacuum Control.vi"("Fill Cutoff Pressure"=w540, "Manifold Pressure"=w544, "Fill State"=T2."Tube Vacuum" ("Current State 2"), "Hold State"=T2."Fill Hold" ("Current State 2")) -> ("Valve Open?"=w547:bool, "Output State"=w536:T2)  [unwired: 6 in]
                      n284 = Wait (ms)(milliseconds to wait=w534) -> ()  [unwired: 1 out]
                      n285 = Equal?(x=w536, y=w535) -> (x = y?=w537:bool)
                      n286 = Absolute Value(x=w555) -> (abs(x)=w558:dbl[unit])
                      n287 = Build Array (concatenate)(w548, w547) -> (w560:bool[])
                      n288 = case shown="False" w537 {
                        tunnel: w543 -> [w570 _]
                        tunnel: w542 -> [w569 _]
                        tunnel: w536 -> [w564 _]
                        frame False {
                          n289 = local read "valve\nrefs"() -> (w571:refnum<vi>[])
                          n290 = control-ref of="Tube State"() -> (w566:refnum<vi>)
                          n291 = call "Set Tube State.vi"("State"=w564, "valve refs"=w571, "error in"=w569, "tube state ref"=w566, "task in"=w570) -> ("error out"=w567:errorcluster)  [unwired: 3 in, 1 out]
                          n292 = Equal?(x=w564, y=T2."Tube Vacuum" ("Current State 2")) -> (x = y?=w568:bool)
                          n293 = case "Wait 5 second if new state is vacuum" shown="True" w568 {
                            tunnel: w567 -> [_ _]
                            frame False {
                            }
                            frame True {
                              n294 = Get Date/Time In Seconds() -> (seconds since 1Jan1904=w573:timestamp)
                              n295 = To Double Precision Float(number=w573) -> (double precision float=w572:dbl)
                              n296 = while {
                                tunnel: w572 -> [w579]
                                stop <- w574 stop-if-true
                                n297 = Get Date/Time In Seconds() -> (seconds since 1Jan1904=w581:timestamp)
                                n298 = To Double Precision Float(number=w581) -> (double precision float=w580:dbl)
                                n299 = Subtract(x=w580, y=w579) -> (x-y=w578:dbl)
                                n300 = Less Or Equal?(x=5.0, y=w578) -> (x <= y?=w576:bool)
                                n301 = local read "Stop"() -> (w575:bool)
                                n302 = Or(x=w576, y=w575) -> (x .or. y?=w574:bool)
                              }
                            }
                          }
                        }
                        frame True {
                        }
                      }
                      n303 = Divide(x=w558, y=w539) -> (x/y=w557:dbl)
                      n304 = Boolean To (0,1)(Boolean=w560) -> (0, 1=w549:i16[])
                      n305 = To Double Precision Float(number=w549) -> (double precision float=w550:dbl[])
                      n306 = Multiply(x=100.0, y=w557) -> (x*y=→"vac err":dbl)
                      n307 = call-poly <vilib>:"Mean.vi"("X"=w550) -> ("mean"=w551:dbl)  [unwired: 1 out]
                      n308 = Less?(x=w551, y=w559) -> (x < y?=w554:bool)
                      n309 = local read "Stop"() -> (w553:bool)
                      n310 = Or(x=w554, y=w553) -> (x .or. y?=w541:bool)
                    }
                    n311 = disable-structure "Log vacuum pressure" shown="Default" {
                      disable-tunnel: w482 -> [_]
                      frame Enabled {
                        w494 = dbl[] []
                        n312 = local read "Sensor sample period (ms)"() -> (w496:i32)
                        n313 = Get Date/Time In Seconds() -> (seconds since 1Jan1904=w498:timestamp)
                        n314 = local read "Pressure measure time"() -> (w499:dbl[unit])
                        n315 = To Double Precision Float(number=w498) -> (double precision float=w495:dbl)
                        n316 = node(w499) -> (w492:dbl)
                        n317 = To Unsigned Long Integer(number=w496) -> (unsigned 32bit integer=w491:u32)
                        n318 = while {
                          shift-right: [w529] -> w503
                          shift-left: w494 -> [w528]
                          tunnel: w491 -> [w526]
                          tunnel: w495 -> [w525]
                          tunnel: w492 -> [w515]
                          shift-right: [w522] -> w502
                          shift-left: timestamp[] [] ("seconds since 1Jan1904") -> [w523]
                          shift-right: [w519] -> w501
                          shift-left: w494 -> [w518]
                          stop <- w517 stop-if-true
                          n319 = Wait (ms)(milliseconds to wait=w526) -> ()  [unwired: 1 out]
                          n320 = Get Date/Time In Seconds() -> (seconds since 1Jan1904=w524:timestamp)
                          n321 = local read "Manifold Pressure"() -> (w530:dbl[unit])
                          n322 = local read "Manifold Temp"() -> (w521:dbl[unit])
                          n323 = To Double Precision Float(number=w524) -> (double precision float=w533:dbl)
                          n324 = Build Array (concatenate)(w523, w524) -> (w522:timestamp[])
                          n325 = Subtract(x=w533, y=w525) -> (x-y=w532:dbl)
                          n326 = local read "Stop"() -> (w516:bool)
                          n327 = Greater Or Equal?(x=w532, y=w515) -> (x >= y?=w531:bool)
                          n328 = node(w530) -> (w527:dbl)
                          n329 = node(w521) -> (w520:dbl)
                          n330 = Or(x=w531, y=w516) -> (x .or. y?=w517:bool)
                          n331 = Build Array (concatenate)(w518, w520) -> (w519:dbl[])
                          n332 = Build Array (concatenate)(w528, w527) -> (w529:dbl[])
                        }
                        "log_vac_press" <- w503
                        "log_vac_time" <- w502
                        "log_vac_temp" <- w501
                        n333 = local read "Fuel Cutoff (default)"() -> (w511:dbl[unit])
                        n334 = local read "Vacuum Cutoff"() -> (w493:dbl[unit])
                        n335 = local read "Diluent Cutoff (default)"() -> (w512:dbl[unit])
                        n336 = local read "Vacuum Cutoff"() -> (w490:dbl[unit])
                        n337 = call-poly <vilib>:"Mean.vi"("X"=w503) -> ("mean"=w513:dbl)  [unwired: 1 out]
                        n338 = node(w513) -> (w514:dbl[unit])
                        "Vacuum Cutoff (actual)" <- w514
                        n339 = Subtract(x=w514, y=w490) -> (x-y=w507:dbl[unit])
                        n340 = Subtract(x=w514, y=w493) -> (x-y=w508:dbl[unit])
                        n341 = Add(x=w508, y=w511) -> (x+y=w510:dbl[unit])
                        n342 = Add(x=w508, y=w512) -> (x+y=w509:dbl[unit])
                        n343 = Absolute Value(x=w507) -> (abs(x)=w505:dbl[unit])
                        n344 = Divide(x=w505, y=w490) -> (x/y=w506:dbl)
                        n345 = local write "Diluent Cutoff (adjusted)"(w509) -> ()
                        n346 = local write "Fuel Cutoff (adjusted)"(w510) -> ()
                        n347 = Multiply(x=100.0, y=w506) -> (x*y=w504:dbl)
                        n348 = local write "vac err"(w504) -> ()
                      }
                    }
                  }
                  frame True {
                  }
                }
              }
              frame #5 {
                # "Fuel Fill"
                n349 = local read "Stop"() -> (w584:bool)
                n350 = case shown="False" w584 {
                  tunnel: w586 -> [w596 _]
                  tunnel: w585 -> [w595 _]
                  tunnel: w583 -> [w591 _]
                  tunnel: w582 -> [w589 _]
                  frame False {
                    n351 = Decrement(x=w591) -> (x-1=w590:i32)
                    n352 = To Double Precision Float(number=w591) -> (double precision float=w594:dbl)
                    n353 = Reciprocal(x=w594) -> (1/x=w593:dbl)
                    n354 = local read "Sensor sample period (ms)"() -> (w588:i32)
                    n355 = To Unsigned Long Integer(number=w588) -> (unsigned 32bit integer=w587:u32)
                    n356 = while {
                      shift-right: [w661] -> _
                      shift-left: w589 -> [w667]
                      tunnel: w593 -> [w660]
                      tunnel: w596 -> [w644]
                      tunnel: w595 -> [w643]
                      tunnel: [w646] -> w592
                      tunnel: w590 -> [w645]
                      tunnel: w587 -> [w642]
                      shift-right: [w640] -> _
                      shift-left: _ -> [w639]
                      stop <- w646 stop-if-true
                      # "Fuel fill"
                      n357 = local read "Fuel Cutoff (adjusted)"() -> (w649:dbl[unit])
                      n358 = Array Subset(array=w667, index=1, length=w645) -> (w663:bool[])
                      n359 = local read "Manifold Pressure"() -> (w650:dbl[unit])
                      n360 = Subtract(x=w649, y="Fuel underpressure") -> (x-y=w647:dbl[unit])
                      n361 = Wait (ms)(milliseconds to wait=w642) -> ()  [unwired: 1 out]
                      n362 = Subtract(x=w650, y=w647) -> (x-y=w658:dbl[unit])
                      n363 = call "Fill Control.vi"("Fill Cutoff Pressure"=w647, "Manifold Pressure"=w650, "Fill State"=T2."Fuel Fill" ("Current State 2"), "Hold State"=T2."Fill Hold" ("Current State 2")) -> ("Valve Open?"=w662:bool, "Output State"=w640:T2)  [unwired: 6 in]
                      n364 = Equal?(x=w640, y=w639) -> (x = y?=w641:bool)
                      n365 = case shown="False" w641 {
                        tunnel: w644 -> [w673 _]
                        tunnel: w643 -> [w672 _]
                        tunnel: w640 -> [w669 _]
                        frame False {
                          n366 = local read "valve\nrefs"() -> (w671:refnum<vi>[])
                          n367 = control-ref of="Tube State"() -> (w670:refnum<vi>)
                          n368 = call "Set Tube State.vi"("State"=w669, "valve refs"=w671, "error in"=w672, "tube state ref"=w670, "task in"=w673) -> ()  [unwired: 3 in, 2 out]
                        }
                        frame True {
                        }
                      }
                      n369 = Build Array (concatenate)(w663, w662) -> (w661:bool[])
                      n370 = Absolute Value(x=w658) -> (abs(x)=w659:dbl[unit])
                      n371 = Divide(x=w659, y=w647) -> (x/y=w654:dbl)
                      n372 = Boolean To (0,1)(Boolean=w661) -> (0, 1=w664:i16[])
                      n373 = To Double Precision Float(number=w664) -> (double precision float=w665:dbl[])
                      n374 = Multiply(x=100.0, y=w654) -> (x*y=→"fuel err":dbl)
                      n375 = call-poly <vilib>:"Mean.vi"("X"=w665) -> ("mean"=w666:dbl)  [unwired: 1 out]
                      n376 = Less?(x=w666, y=w660) -> (x < y?=w652:bool)
                      n377 = local read "Stop"() -> (w651:bool)
                      n378 = Or(x=w652, y=w651) -> (x .or. y?=w646:bool)
                    }
                    n379 = disable-structure "Log fill pressure" shown="Default" {
                      disable-tunnel: w592 -> [_]
                      frame Enabled {
                        w602 = dbl[] []
                        n380 = local read "Pressure measure time"() -> (w601:dbl[unit])
                        n381 = local read "Sensor sample period (ms)"() -> (w604:i32)
                        n382 = Get Date/Time In Seconds() -> (seconds since 1Jan1904=w600:timestamp)
                        n383 = To Double Precision Float(number=w600) -> (double precision float=w599:dbl)
                        n384 = node(w601) -> (w598:dbl)
                        n385 = To Unsigned Long Integer(number=w604) -> (unsigned 32bit integer=w597:u32)
                        n386 = while {
                          tunnel: w599 -> [w637]
                          tunnel: w597 -> [w636]
                          tunnel: w598 -> [w620]
                          shift-right: [w632] -> w619
                          shift-left: w602 -> [w631]
                          shift-right: [w627] -> w607
                          shift-left: timestamp[] [] ("seconds since 1Jan1904") -> [w628]
                          shift-right: [w624] -> w606
                          shift-left: w602 -> [w623]
                          stop <- w622 stop-if-true
                          n387 = Wait (ms)(milliseconds to wait=w636) -> ()  [unwired: 1 out]
                          n388 = Get Date/Time In Seconds() -> (seconds since 1Jan1904=w629:timestamp)
                          n389 = local read "Manifold Pressure"() -> (w633:dbl[unit])
                          n390 = local read "Manifold Temp"() -> (w625:dbl[unit])
                          n391 = To Double Precision Float(number=w629) -> (double precision float=w638:dbl)
                          n392 = Build Array (concatenate)(w628, w629) -> (w627:timestamp[])
                          n393 = Subtract(x=w638, y=w637) -> (x-y=w635:dbl)
                          n394 = local read "Stop"() -> (w621:bool)
                          n395 = node(w633) -> (w630:dbl)
                          n396 = Greater Or Equal?(x=w635, y=w620) -> (x >= y?=w634:bool)
                          n397 = node(w625) -> (w626:dbl)
                          n398 = Or(x=w621, y=w634) -> (x .or. y?=w622:bool)
                          n399 = Build Array (concatenate)(w631, w630) -> (w632:dbl[])
                          n400 = Build Array (concatenate)(w623, w626) -> (w624:dbl[])
                        }
                        "log_fuel_press" <- w619
                        "log_fuel_time" <- w607
                        "log_fuel_temp" <- w606
                        n401 = local read "Fuel Cutoff (adjusted)"() -> (w610:dbl[unit])
                        n402 = local read "Fuel Cutoff (adjusted)"() -> (w617:dbl[unit])
                        n403 = local read "Diluent Cutoff (adjusted)"() -> (w616:dbl[unit])
                        n404 = call-poly <vilib>:"Mean.vi"("X"=w619) -> ("mean"=w618:dbl)  [unwired: 1 out]
                        n405 = node(w618) -> (w609:dbl[unit])
                        "Fuel Cutoff (actual)" <- w609
                        n406 = Subtract(x=w609, y=w610) -> (x-y=w612:dbl[unit])
                        n407 = Subtract(x=w609, y=w617) -> (x-y=w615:dbl[unit])
                        n408 = Add(x=w616, y=w615) -> (x+y=w614:dbl[unit])
                        n409 = Absolute Value(x=w612) -> (abs(x)=w613:dbl[unit])
                        n410 = Divide(x=w613, y=w610) -> (x/y=w611:dbl)
                        n411 = local write "Diluent Cutoff (adjusted)"(w614) -> ()
                        n412 = Multiply(x=100.0, y=w611) -> (x*y=w608:dbl)
                        n413 = local write "fuel err"(w608) -> ()
                      }
                    }
                  }
                  frame True {
                  }
                }
              }
              frame #6 {
                # "Diluent Fill"
                n414 = local read "Stop"() -> (w676:bool)
                n415 = case shown="False" w676 {
                  tunnel: w678 -> [w685 _]
                  tunnel: w677 -> [w684 _]
                  tunnel: w675 -> [w687 _]
                  tunnel: w674 -> [w686 _]
                  frame False {
                    n416 = local read "Diluent Cutoff (default)"() -> (w697:dbl[unit])
                    n417 = local read "Fuel Cutoff (default)"() -> (w696:dbl[unit])
                    n418 = local read "Diluent"() -> (w694:string)
                    n419 = To Double Precision Float(number=w687) -> (double precision float=w689:dbl)
                    n420 = Equal?(x=w694, y="") -> (x = y?=w693:bool)
                    n421 = Reciprocal(x=w689) -> (1/x=w688:dbl)
                    n422 = Greater?(x=w697, y=w696) -> (0:w695:bool)
                    n423 = Not(x=w693) -> (.not. x?=w691:bool)
                    n424 = Or(x=w695, y=w691) -> (x .or. y?=w692:bool)
                    "is diluted?" <- w692
                    n425 = case shown="True" w692 {
                      tunnel: w686 -> [_ w725]
                      tunnel: w687 -> [_ w722]
                      tunnel: w688 -> [_ w724]
                      tunnel: w685 -> [_ w721]
                      tunnel: w684 -> [_ w720]
                      tunnel: [w700 w712] -> w683
                      tunnel: [w700 w710] -> w682
                      tunnel: [w699 w711] -> w681
                      tunnel: timestamp[] [] ("seconds since 1Jan1904") -> [w699 w709]
                      tunnel: dbl[] [] -> [w700 w708]
                      frame False {
                        n426 = local read "Fuel Cutoff (actual)"() -> (w698:dbl[unit])
                        n427 = local write "Diluent Cutoff (actual)"(w698) -> ()
                      }
                      frame True {
                        n428 = Decrement(x=w722) -> (x-1=w723:i32)
                        n429 = while {
                          shift-right: [w768] -> _
                          shift-left: w725 -> [w774]
                          tunnel: w724 -> [w767]
                          tunnel: w723 -> [w755]
                          tunnel: w721 -> [w753]
                          tunnel: w720 -> [w752]
                          tunnel: [w754] -> w706
                          shift-right: [w748] -> _
                          shift-left: _ -> [w747]
                          stop <- w754 stop-if-true
                          n430 = local read "Diluent Cutoff (adjusted)"() -> (w757:dbl[unit])
                          n431 = Array Subset(array=w774, index=1, length=w755) -> (w770:bool[])
                          n432 = local read "Manifold Pressure"() -> (w758:dbl[unit])
                          n433 = Subtract(x=w757, y="Diluent underpressure") -> (x-y=w756:dbl[unit])
                          n434 = Subtract(x=w758, y=w756) -> (x-y=w765:dbl[unit])
                          n435 = call "Fill Control.vi"("Fill Cutoff Pressure"=w756, "Manifold Pressure"=w758, "Fill State"=T2."Diluent Fill" ("Current State 2"), "Hold State"=T2."Fill Hold" ("Current State 2")) -> ("Valve Open?"=w769:bool, "Output State"=w748:T2)  [unwired: 6 in]
                          n436 = Absolute Value(x=w765) -> (abs(x)=w766:dbl[unit])
                          n437 = Build Array (concatenate)(w770, w769) -> (w768:bool[])
                          n438 = Boolean To (0,1)(Boolean=w768) -> (0, 1=w771:i16[])
                          n439 = Divide(x=w766, y=w756) -> (x/y=w762:dbl)
                          n440 = Equal?(x=w748, y=w747) -> (x = y?=w749:bool)
                          n441 = To Double Precision Float(number=w771) -> (double precision float=w772:dbl[])
                          n442 = Multiply(x=100.0, y=w762) -> (x*y=→"dil err":dbl)
                          n443 = case shown="False" w749 {
                            tunnel: w748 -> [w780 _]
                            tunnel: w753 -> [w778 _]
                            tunnel: w752 -> [w777 _]
                            frame False {
                              n444 = local read "valve\nrefs"() -> (w779:refnum<vi>[])
                              n445 = control-ref of="Tube State"() -> (w776:refnum<vi>)
                              n446 = call "Set Tube State.vi"("State"=w780, "valve refs"=w779, "error in"=w777, "tube state ref"=w776, "task in"=w778) -> ()  [unwired: 3 in, 2 out]
                            }
                            frame True {
                            }
                          }
                          n447 = call-poly <vilib>:"Mean.vi"("X"=w772) -> ("mean"=w773:dbl)  [unwired: 1 out]
                          n448 = Less?(x=w773, y=w767) -> (x < y?=w760:bool)
                          n449 = local read "Stop"() -> (w759:bool)
                          n450 = Or(x=w760, y=w759) -> (x .or. y?=w754:bool)
                        }
                        n451 = local read "Sensor sample period (ms)"() -> (w705:i32)
                        n452 = local read "Pressure measure time"() -> (w704:dbl[unit])
                        n453 = disable-structure shown="Default" {
                          disable-tunnel: [w726] -> w707
                          disable-tunnel: w706 -> [_]
                          frame Enabled {
                            n454 = Get Date/Time In Seconds() -> (seconds since 1Jan1904=w727:timestamp)
                            n455 = To Double Precision Float(number=w727) -> (double precision float=w726:dbl)
                          }
                        }
                        n456 = To Unsigned Long Integer(number=w705) -> (unsigned 32bit integer=w701:u32)
                        n457 = node(w704) -> (w702:dbl)
                        n458 = while {
                          shift-right: [w742] -> w712
                          shift-left: w708 -> [w741]
                          shift-right: [w738] -> w711
                          shift-left: w709 -> [w737]
                          shift-right: [w733] -> w710
                          shift-left: w708 -> [w734]
                          tunnel: w702 -> [w728]
                          tunnel: w707 -> [w730]
                          tunnel: w701 -> [w729]
                          stop <- w732 stop-if-true
                          n459 = Wait (ms)(milliseconds to wait=w729) -> ()  [unwired: 1 out]
                          n460 = Get Date/Time In Seconds() -> (seconds since 1Jan1904=w739:timestamp)
                          n461 = local read "Manifold Pressure"() -> (w743:dbl[unit])
                          n462 = local read "Manifold Temp"() -> (w736:dbl[unit])
                          n463 = To Double Precision Float(number=w739) -> (double precision float=w746:dbl)
                          n464 = Build Array (concatenate)(w737, w739) -> (w738:timestamp[])
                          n465 = Subtract(x=w746, y=w730) -> (x-y=w745:dbl)
                          n466 = node(w743) -> (w740:dbl)
                          n467 = Greater Or Equal?(x=w745, y=w728) -> (x >= y?=w744:bool)
                          n468 = node(w736) -> (w735:dbl)
                          n469 = local read "Stop"() -> (w731:bool)
                          n470 = Build Array (concatenate)(w734, w735) -> (w733:dbl[])
                          n471 = Build Array (concatenate)(w741, w740) -> (w742:dbl[])
                          n472 = Or(x=w731, y=w744) -> (x .or. y?=w732:bool)
                        }
                        n473 = local read "Diluent Cutoff (adjusted)"() -> (w718:dbl[unit])
                        n474 = call-poly <vilib>:"Mean.vi"("X"=w712) -> ("mean"=w714:dbl)  [unwired: 1 out]
                        n475 = node(w714) -> (w703:dbl[unit])
                        "Diluent Cutoff (actual)" <- w703
                        n476 = Subtract(x=w703, y=w718) -> (x-y=w716:dbl[unit])
                        n477 = Absolute Value(x=w716) -> (abs(x)=w717:dbl[unit])
                        n478 = Divide(x=w717, y=w718) -> (x/y=w715:dbl)
                        n479 = Multiply(x=100.0, y=w715) -> (x*y=w719:dbl)
                        n480 = local write "dil err"(w719) -> ()
                      }
                    }
                    "log_dil_press" <- w683
                    "log_dil_time" <- w681
                    "log_dil_temp" <- w682
                  }
                  frame True {
                  }
                }
              }
              frame #7 {
                # "Oxidizer Fill"
                n481 = local read "Stop"() -> (w783:bool)
                n482 = case shown="False" w783 {
                  tunnel: w785 -> [w791 _]
                  tunnel: w784 -> [w790 _]
                  tunnel: w782 -> [w793 _]
                  tunnel: w781 -> [w788 _]
                  frame False {
                    n483 = Decrement(x=w793) -> (x-1=w789:i32)
                    n484 = To Double Precision Float(number=w793) -> (double precision float=w794:dbl)
                    n485 = local read "Sensor sample period (ms)"() -> (w787:i32)
                    n486 = Reciprocal(x=w794) -> (1/x=w795:dbl)
                    n487 = To Unsigned Long Integer(number=w787) -> (unsigned 32bit integer=w786:u32)
                    n488 = while {
                      shift-right: [w816] -> _
                      shift-left: w788 -> [w822]
                      tunnel: w795 -> [w815]
                      tunnel: [w803] -> w792
                      tunnel: w791 -> [w802]
                      tunnel: w790 -> [w800]
                      tunnel: w789 -> [w801]
                      shift-right: [w798] -> _
                      shift-left: _ -> [w797]
                      tunnel: w786 -> [w796]
                      stop <- w806 stop-if-true
                      n489 = local read "Oxidizer Cutoff (default)"() -> (w812:dbl[unit])
                      n490 = Array Subset(array=w822, index=1, length=w801) -> (w818:bool[])
                      n491 = local read "Manifold Pressure"() -> (w805:dbl[unit])
                      n492 = Wait (ms)(milliseconds to wait=w796) -> ()  [unwired: 1 out]
                      n493 = Subtract(x=w805, y=w812) -> (x-y=w813:dbl[unit])
                      n494 = call "Fill Control.vi"("Fill Cutoff Pressure"=w812, "Manifold Pressure"=w805, "Fill State"=T2."Oxidizer Fill" ("Current State 2"), "Hold State"=T2."Fill Hold" ("Current State 2")) -> ("Valve Open?"=w817:bool, "Output State"=w798:T2)  [unwired: 6 in]
                      n495 = Absolute Value(x=w813) -> (abs(x)=w814:dbl[unit])
                      n496 = Build Array (concatenate)(w818, w817) -> (w816:bool[])
                      n497 = Equal?(x=w798, y=w797) -> (x = y?=w799:bool)
                      n498 = Boolean To (0,1)(Boolean=w816) -> (0, 1=w819:i16[])
                      n499 = Divide(x=w814, y=w812) -> (x/y=w809:dbl)
                      n500 = case shown="False" w799 {
                        tunnel: w802 -> [w828 _]
                        tunnel: w798 -> [w827 _]
                        tunnel: w800 -> [w826 _]
                        frame False {
                          n501 = control-ref of="Tube State"() -> (w824:refnum<vi>)
                          n502 = local read "valve\nrefs"() -> (w825:refnum<vi>[])
                          n503 = call "Set Tube State.vi"("State"=w827, "valve refs"=w825, "error in"=w826, "tube state ref"=w824, "task in"=w828) -> ()  [unwired: 3 in, 2 out]
                        }
                        frame True {
                        }
                      }
                      n504 = To Double Precision Float(number=w819) -> (double precision float=w820:dbl[])
                      n505 = Multiply(x=100.0, y=w809) -> (x*y=→"ox err":dbl)
                      n506 = call-poly <vilib>:"Mean.vi"("X"=w820) -> ("mean"=w821:dbl)  [unwired: 1 out]
                      n507 = local read "Stop"() -> (w803:bool)
                      n508 = Less?(x=w821, y=w815) -> (x < y?=w807:bool)
                      n509 = Or(x=w807, y=w803) -> (x .or. y?=w806:bool)
                    }
                    n510 = disable-structure shown="Default" {
                      disable-tunnel: w792 -> [_]
                      frame Enabled {
                        # "if oxidizer is air, add vacuum pressure because that's air too"
                        n511 = local read "Sensor sample period (ms)"() -> (w833:i32)
                        n512 = local read "Pressure measure time"() -> (w836:dbl[unit])
                        n513 = Get Date/Time In Seconds() -> (seconds since 1Jan1904=w835:timestamp)
                        n514 = To Double Precision Float(number=w835) -> (double precision float=w832:dbl)
                        n515 = To Unsigned Long Integer(number=w833) -> (unsigned 32bit integer=w829:u32)
                        n516 = node(w836) -> (w830:dbl)
                        n517 = while {
                          tunnel: w832 -> [w882]
                          tunnel: w830 -> [w865]
                          shift-right: [w878] -> w863
                          shift-left: _ -> [w877]
                          shift-right: [w874] -> w840
                          shift-left: timestamp[] [] ("seconds since 1Jan1904") -> [w873]
                          shift-right: [w869] -> w839
                          shift-left: dbl[] [] -> [w870]
                          tunnel: w829 -> [w868]
                          stop <- w867 stop-if-true
                          n518 = Wait (ms)(milliseconds to wait=w868) -> ()  [unwired: 1 out]
                          n519 = Get Date/Time In Seconds() -> (seconds since 1Jan1904=w875:timestamp)
                          n520 = local read "Manifold Pressure"() -> (w879:dbl[unit])
                          n521 = local read "Manifold Temp"() -> (w872:dbl[unit])
                          n522 = To Double Precision Float(number=w875) -> (double precision float=w883:dbl)
                          n523 = Build Array (concatenate)(w873, w875) -> (w874:timestamp[])
                          n524 = Subtract(x=w883, y=w882) -> (x-y=w881:dbl)
                          n525 = local read "Stop"() -> (w866:bool)
                          n526 = node(w879) -> (w876:dbl)
                          n527 = Greater Or Equal?(x=w881, y=w865) -> (x >= y?=w880:bool)
                          n528 = node(w872) -> (w871:dbl)
                          n529 = Or(x=w866, y=w880) -> (x .or. y?=w867:bool)
                          n530 = Build Array (concatenate)(w870, w871) -> (w869:dbl[])
                          n531 = Build Array (concatenate)(w877, w876) -> (w878:dbl[])
                        }
                        "log_ox_press" <- w863
                        "log_ox_time" <- w840
                        "log_ox_temp" <- w839
                        n532 = local read "Diluent Cutoff (actual)"() -> (w842:dbl[unit])
                        n533 = local read "Oxidizer"() -> (w862:string)
                        n534 = local read "Fuel Cutoff (actual)"() -> (w843:dbl[unit])
                        n535 = local read "Oxidizer Cutoff (default)"() -> (w848:dbl[unit])
                        n536 = local read "Diluent Cutoff (actual)"() -> (w858:dbl[unit])
                        n537 = local read "Vacuum Cutoff (actual)"() -> (w841:dbl[unit])
                        n538 = Subtract(x=w842, y=w843) -> (x-y=w844:dbl[unit])
                        n539 = call-poly <vilib>:"Mean.vi"("X"=w863) -> ("mean"=w864:dbl)  [unwired: 1 out]
                        n540 = node(w864) -> (w845:dbl[unit])
                        "Oxidizer Cutoff (actual)" <- w845
                        n541 = Divide(x=w844, y=w845) -> (x/y=→"dil_mf_measured":dbl)
                        n542 = Subtract(x=w845, y=w848) -> (x-y=w849:dbl[unit])
                        n543 = Subtract(x=w845, y=w858) -> (x-y=w857:dbl[unit])
                        n544 = To Lower Case(string=w862) -> (all lower case string=w861:string)
                        n545 = Absolute Value(x=w849) -> (abs(x)=w850:dbl[unit])
                        n546 = Add(x=w857, y=w841) -> (x+y=w859:dbl[unit])
                        n547 = Subtract(x=w843, y=w841) -> (x-y=w856:dbl[unit])
                        n548 = Equal?(x="air", y=w861) -> (x = y?=w860:bool)
                        n549 = Divide(x=w850, y=w848) -> (x/y=w847:dbl)
                        n550 = Select(t=w859, s=w860, f=w857) -> (s? t:f=w855:dbl[unit])
                        n551 = Divide(x=w856, y=w855) -> (x/y=w854:dbl)
                        n552 = local read "f_a_st"() -> (w853:dbl)
                        n553 = Multiply(x=100.0, y=w847) -> (x*y=w851:dbl)
                        n554 = local write "ox err"(w851) -> ()
                        n555 = Divide(x=w854, y=w853) -> (x/y=→"phi actual":dbl)
                      }
                    }
                  }
                  frame True {
                  }
                }
              }
              frame #8 {
                # "Mix"
                n556 = local read "Stop"() -> (w884:bool)
                n557 = case shown="False" w884 {
                  tunnel: w886 -> [w899 _]
                  tunnel: w885 -> [w898 _]
                  frame False {
                    n558 = local read "valve\nrefs"() -> (w887:refnum<vi>[])
                    n559 = control-ref of="Tube State"() -> (w888:refnum<vi>)
                    n560 = call "Set Tube State.vi"("State"=T2."Tube Closed", "valve refs"=w887, "error in"=w898, "tube state ref"=w888, "task in"=w899) -> ("error out"=w897:errorcluster, "task out"=w895:refnum<k21>)  [unwired: 3 in]
                    n561 = call "Wait Valve Actuate.vi"("error in"=w897) -> ("error out"=w896:errorcluster)
                    n562 = call "Set Tube State.vi"("State"=T2."Mixing", "valve refs"=w887, "error in"=w896, "tube state ref"=w888, "task in"=w895) -> ("error out"=w892:errorcluster, "task out"=w889:refnum<k21>)  [unwired: 3 in]
                    n563 = disable-structure shown="Default" {
                      disable-tunnel: [w912] -> w903
                      disable-tunnel: w892 -> [w911]
                      disable-tunnel: [w911] -> w890
                      frame Enabled {
                        n564 = Get Date/Time In Seconds() -> (seconds since 1Jan1904=w912:timestamp)
                      }
                    }
                    n565 = To Double Precision Float(number=w903) -> (double precision float=w891:dbl)
                    n566 = node("Mix Time") -> (w902:dbl)
                    n567 = while {
                      tunnel: w891 -> [w920]
                      tunnel: w902 -> [w916]
                      tunnel: [w917] -> w900
                      stop <- w917 stop-if-true
                      n568 = Get Date/Time In Seconds() -> (seconds since 1Jan1904=w921:timestamp)
                      n569 = To Double Precision Float(number=w921) -> (double precision float=w913:dbl)
                      n570 = Subtract(x=w913, y=w920) -> (x-y=w915:dbl)
                      n571 = local read "Stop"() -> (w918:bool)
                      n572 = Subtract(x=w916, y=w915) -> (x-y=w914:dbl)
                      n573 = Less Or Equal?(x=w916, y=w915) -> (x <= y?=w919:bool)
                      n574 = Or(x=w919, y=w918) -> (x .or. y?=w917:bool)
                      n575 = local write "Remaining"(w914) -> ()
                    }
                    n576 = disable-structure shown="Default" {
                      disable-tunnel: w900 -> [_]
                      disable-tunnel: w890 -> [w908]
                      disable-tunnel: w889 -> [w907]
                      disable-tunnel: w888 -> [w906]
                      disable-tunnel: w887 -> [w904]
                      frame Enabled {
                        n577 = local write "Remaining"(0.0 ("Remaining")) -> ()
                        n578 = call "Set Tube State.vi"("State"=T2."Tube Closed", "valve refs"=w904, "error in"=w908, "tube state ref"=w906, "task in"=w907) -> ("error out"=w909:errorcluster)  [unwired: 3 in, 1 out]
                        n579 = call "Wait Valve Actuate.vi"("error in"=w909) -> ()  [unwired: 1 out]
                      }
                    }
                  }
                  frame True {
                  }
                }
              }
              frame #9 {
                # "Detonate"
                n580 = local read "Stop"() -> (w922:bool)
                n581 = case shown="False" w922 {
                  tunnel: w926 -> [w930 _]
                  tunnel: w925 -> [w929 _]
                  tunnel: w924 -> [w928 _]
                  tunnel: [w927 _] -> w923
                  frame False {
                    n582 = call "Make Shot Directory.vi"("daily test directory"=w930) -> ("shot directory"=w927:path)  [unwired: 8 in, 1 out]
                    n583 = disable-structure "Diode control and logging" shown="Default" {
                      disable-tunnel: w927 -> [w943]
                      disable-tunnel: w929 -> [w938]
                      disable-tunnel: w928 -> [w937]
                      frame Enabled {
                        w940 = u32 100  # Ignition event time
                        w941 = u32 5  # Ignition high time (ms)
                        w939 = 10  # Number of spark pulses
                        n584 = Build Path(base path=w943, name or relative path="diodes.tdms") -> (appended path=w936:path)
                        n585 = call "Read Photodiodes.vi"("Diode tdms path"=w936) -> ("error out"=w945:errorcluster)  [unwired: 3 in]
                        n586 = call <vilib>:"Clear Errors.vi"("error in (no error)"=w945) -> ()  [unwired: 5 in, 2 out]
                        n587 = case shown="No Error" w945 {
                          tunnel: [u32 6618880 ("Text.Text Colors:BG Color") u32 16711680 ("Text.Text Colors:BG Color")] -> w933
                          tunnel: ["Diode read OK" "Diode read BAD"] -> w934
                          frame No Error {
                          }
                          frame Error {
                          }
                        }
                        n588 = disable-structure "100 ms wait to ensure logging has time to initiate" shown="Default" {
                          disable-tunnel: w936 -> [_]
                          disable-tunnel: [w946] -> w935
                          frame Enabled {
                            n589 = Wait (ms)(milliseconds to wait=u32 100) -> (millisecond timer value=w946:u32)
                          }
                        }
                        n590 = local write "diode read status"(w934) -> ()
                        n591 = property on="diode read status" class="Str"("Text.BGColor"=w933) -> ()  [unwired: 2 in, 2 out]
                        n592 = Subtract(x=w940, y=w941) -> (x-y=w942:u32)
                        n593 = control-ref of="Tube State"() -> (w931:refnum<vi>)
                        n594 = for "Send spark signal" {
                          N: w939 -> [_]
                          tunnel: w941 -> [w957]
                          tunnel: w942 -> [w956]
                          tunnel: w938 -> [w951]
                          shift-right: [w952] -> w932
                          shift-left: w937 -> [w950]
                          tunnel: w935 -> [_]
                          tunnel: w931 -> [w948]
                          n595 = disable-structure "Pulse ON" shown="Default" {
                            disable-tunnel: w957 -> [w973]
                            disable-tunnel: [w972] -> w955
                            disable-tunnel: [w968] -> w954
                            disable-tunnel: [w967] -> w953
                            disable-tunnel: w951 -> [w970]
                            disable-tunnel: w950 -> [w969]
                            disable-tunnel: [w966] -> w949
                            disable-tunnel: w948 -> [w965]
                            frame Enabled {
                              n596 = Wait (ms)(milliseconds to wait=w973) -> (millisecond timer value=w972:u32)
                              n597 = local read "valve\nrefs"() -> (w966:refnum<vi>[])
                              n598 = call "Set Tube State.vi"("State"=T2."Ignition", "valve refs"=w966, "error in"=w969, "tube state ref"=w965, "task in"=w970) -> ("error out"=w967:errorcluster, "task out"=w968:refnum<k21>)  [unwired: 3 in]
                            }
                          }
                          n599 = disable-structure "Pulse OFF" shown="Default" {
                            disable-tunnel: w956 -> [w964]
                            disable-tunnel: w955 -> [_]
                            disable-tunnel: w954 -> [w962]
                            disable-tunnel: w953 -> [w961]
                            disable-tunnel: [w960] -> w952
                            disable-tunnel: w949 -> [w959]
                            disable-tunnel: w948 -> [w958]
                            frame Enabled {
                              n600 = Wait (ms)(milliseconds to wait=w964) -> ()  [unwired: 1 out]
                              n601 = call "Set Tube State.vi"("State"=T2."Tube Closed", "valve refs"=w959, "error in"=w961, "tube state ref"=w958, "task in"=w962) -> ("error out"=w960:errorcluster)  [unwired: 3 in, 1 out]
                            }
                          }
                        }
                        n602 = call <vilib>:"Simple Error Handler.vi"("error in (no error)"=w932) -> ()  [unwired: 4 in, 5 out]
                      }
                    }
                    n603 = disable-structure "Log fill states" shown="Default" {
                      disable-tunnel: w927 -> [w1004]
                      frame Enabled {
                        n604 = Build Path(base path=w1004, name or relative path="fill.tdms") -> (appended path=w978:path)
                        n605 = local read "log_vac_press"() -> (w999:dbl[])
                        n606 = local read "log_vac_temp"() -> (w1000:dbl[])
                        n607 = local read "log_vac_time"() -> (w1001:timestamp[])
                        n608 = TDMS Open(5:FALSE ("create index file? (T)"), 10:T6."open or create" ("operation (0:open)"), 11:w978) -> (3:w998:refnum<k34>)  [unwired: 4 in, 1 out]
                        n609 = call "Log fill data.vi"("component"="vacuum", "time"=w1001, "temp"=w1000, "press"=w999, "tdms file"=w998) -> ("tdms file out"=w995:refnum<k34>)  [unwired: 6 in]
                        n610 = local read "log_fuel_press"() -> (w994:dbl[])
                        n611 = local read "log_fuel_temp"() -> (w996:dbl[])
                        n612 = local read "log_fuel_time"() -> (w997:timestamp[])
                        n613 = call "Log fill data.vi"("component"="fuel", "time"=w997, "temp"=w996, "press"=w994, "tdms file"=w995) -> ("tdms file out"=w990:refnum<k34>)  [unwired: 6 in]
                        n614 = local read "log_dil_press"() -> (w993:dbl[])
                        n615 = local read "log_dil_temp"() -> (w992:dbl[])
                        n616 = local read "log_dil_time"() -> (w991:timestamp[])
                        n617 = call "Log fill data.vi"("component"="diluent", "time"=w991, "temp"=w992, "press"=w993, "tdms file"=w990) -> ("tdms file out"=w986:refnum<k34>)  [unwired: 6 in]
                        n618 = local read "log_ox_press"() -> (w989:dbl[])
                        n619 = local read "log_ox_temp"() -> (w988:dbl[])
                        n620 = local read "log_ox_time"() -> (w987:timestamp[])
                        n621 = call "Log fill data.vi"("component"="oxidizer", "time"=w987, "temp"=w988, "press"=w989, "tdms file"=w986) -> ("tdms file out"=w985:refnum<k34>)  [unwired: 6 in]
                        n622 = TDMS Flush(7:w985) -> (0:w1003:errorcluster, 3:w1002:refnum<k34>)  [unwired: 1 in]
                        n623 = TDMS Close(8:w1003, 11:w1002) -> ()  [unwired: 2 out]
                      }
                    }
                  }
                  frame True {
                  }
                }
              }
              frame #10 {
                # "Tube Vent"
                n624 = local read "Stop"() -> (w1011:bool)
                n625 = case shown="False" w1011 {
                  tunnel: w1010 -> [w1056 w1069]
                  tunnel: w1009 -> [w1051 w1068]
                  tunnel: [w1047 w1069] -> w1007
                  tunnel: [w1046 w1068] -> w1008
                  tunnel: w1006 -> [w1045 _]
                  frame False {
                    w1012 = T3."Enabled" ("Disabled")
                    w1020 = "%Y-%m-%d T%H:%M:%S%6u" ("time format string (%c)")
                    n626 = local read "log_manifold_vent_end"() -> (w1021:timestamp)
                    n627 = local read "log_manifold_vent_start"() -> (w1023:timestamp)
                    n628 = local read "valve\nrefs"() -> (w1050:refnum<vi>[])
                    n629 = control-ref of="Tube State"() -> (w1014:refnum<vi>)
                    n630 = call "Set Tube State.vi"("State"=T2."Tube Vent", "valve refs"=w1050, "error in"=w1051, "tube state ref"=w1014, "task in"=w1056) -> ("error out"=w1055:errorcluster, "task out"=w1047:refnum<k21>)  [unwired: 3 in]
                    n631 = call "Wait Valve Actuate.vi"("error in"=w1055) -> ("error out"=w1053:errorcluster)
                    n632 = Format Date/Time String(time format string (%c)=w1020, seconds (now)=w1023, UTC format=TRUE) -> (date/time string=w1019:string)
                    n633 = Format Date/Time String(time format string (%c)=w1020, seconds (now)=w1021, UTC format=TRUE) -> (date/time string=w1018:string)
                    n634 = local read "Oxidizer Cutoff (default)"() -> (w1032:dbl[unit])
                    n635 = disable-structure shown="Default" {
                      disable-tunnel: [w1059] -> w1036
                      disable-tunnel: w1053 -> [w1058]
                      disable-tunnel: [w1058] -> w1046
                      frame Enabled {
                        n636 = Get Date/Time In Seconds() -> (seconds since 1Jan1904=w1059:timestamp)
                      }
                    }
                    "log_end_time" <- w1036
                    n637 = local read "Atmospheric Pressure"() -> (w1017:dbl[unit])
                    n638 = To Double Precision Float(number=w1036) -> (double precision float=w1049:dbl)
                    n639 = local read "log_start_time"() -> (w1038:timestamp)
                    n640 = local read "Diluent Mole Fraction"() -> (w1028:string)
                    n641 = local read "Equivalence Ratio"() -> (w1029:string)
                    n642 = while {
                      tunnel: w1049 -> [w1066]
                      tunnel: 5.0 -> [w1064]
                      tunnel: [w1060] -> w1048
                      stop <- w1060 stop-if-true
                      # "Allow 5 second vent time"
                      n643 = Get Date/Time In Seconds() -> (seconds since 1Jan1904=w1067:timestamp)
                      n644 = To Double Precision Float(number=w1067) -> (double precision float=w1061:dbl)
                      n645 = Subtract(x=w1061, y=w1066) -> (x-y=w1065:dbl)
                      n646 = Greater Or Equal?(x=w1064, y=w1065) -> (x >= y?=w1063:bool)
                      n647 = local read "Stop"() -> (w1062:bool)
                      n648 = Or(x=w1063, y=w1062) -> (x .or. y?=w1060:bool)
                    }
                    n649 = node(w1032) -> (w1031:dbl)
                    n650 = node(w1017) -> (w1016:dbl)
                    n651 = local read "Oxidizer"() -> (w1026:string)
                    n652 = local read "Diluent"() -> (w1025:string)
                    n653 = local read "Fuel"() -> (w1027:string)
                    n654 = Format Date/Time String(time format string (%c)=w1020, seconds (now)=w1038, UTC format=TRUE) -> (date/time string=w1035:string)
                    n655 = Format Date/Time String(time format string (%c)=w1020, seconds (now)=w1036, UTC format=TRUE) -> (date/time string=w1034:string)
                    n656 = Number To Decimal String(number=w1031) -> (decimal integer string=w1030:string)  [unwired: 1 in]
                    n657 = Number To Decimal String(number=w1016) -> (decimal integer string=w1015:string)  [unwired: 1 in]
                    n658 = Build Array(w1035, w1034, w1030, w1029, w1027, w1026, w1025, w1028, w1019, w1018, w1015) -> (w1033:string[])
                    n659 = disable-structure "Test complete alert" shown="Default" {
                      disable-tunnel: w1048 -> [_]
                      frame Enabled {
                        n660 = call <vilib>:"Beep.vi"() -> ()  [unwired: 12 in]
                        n661 = local write "Test Status"("Ready" ("Test Status")) -> ()
                      }
                    }
                    n662 = Build Path(base path=w1045, name or relative path="conditions.csv") -> (appended path=w1041:path)
                    n663 = Build Array(string[] ["start", "end", "p_0_nom", "phi_nom", "fuel", "oxidizer", "diluent", "dil_mf_nom", "vent_start", "vent_end", "atmospheric"], w1033) -> (w1042:string[][])
                    n664 = call-poly <vilib>:"Write Delimited Spreadsheet.vi"("file path (dialog if empty)"=w1041, "2D data"=w1042, "delimiter (\\t)"="," ("delimiter (\\t)")) -> ("error out"=w1013:errorcluster)  [unwired: 11 in, 1 out]
                    n665 = call <vilib>:"Simple Error Handler.vi"("error in (no error)"=w1013) -> ()  [unwired: 4 in, 5 out]
                    n666 = property on="Run Test" class="Bool"(error in=w1013, "DisabledEnum"=w1012) -> ()  [unwired: 1 in, 2 out]
                    n667 = property on="Set Mode" class="Bool (strict)"(error in=w1013, "DisabledEnum"=w1012) -> ()  [unwired: 1 in, 2 out]
                  }
                  frame True {
                  }
                }
              }
            }
          }
          event "Test condition CSV": Value Change {
            n668 = event-data() -> ()  [unwired: 1 in, 1 out]
            n669 = call "Load CSV.vi"("CSV Path"="Test condition CSV") -> ("Header"=w1073:string[], "error out"=w1074:errorcluster, "CSV Array"=w1075:string[][], "indices"=w1076:T1, "Fuel"=w1079:string[], "Oxidizer"=w1078:string[], "Initial Pressure"=w1077:string[], "Equivalence Ratio"=w1080:string[], "Diluent"=w1081:string[], "Diluent Mole Fraction"=w1082:string[])  [unwired: 9 in]
            n670 = case shown="No Error" w1074 {
              tunnel: w1082 -> [w1094 _]
              tunnel: w1081 -> [w1093 _]
              tunnel: w1080 -> [w1092 _]
              tunnel: w1079 -> [w1091 _]
              tunnel: w1078 -> [w1090 _]
              tunnel: w1077 -> [w1089 _]
              tunnel: w1076 -> [w1088 _]
              tunnel: w1075 -> [w1083 _]
              tunnel: w1073 -> [w1084 _]
              frame No Error {
                w1085 = T3."Enabled" ("Disabled")
                w1087 = "" ("Value (Signaling)")
                n671 = local write "Test CSV Header"(w1084) -> ()
                n672 = local write "Test CSV"(w1083) -> ()
                n673 = property on="Fuel" class="CmbBox"("Strings[]"=w1091, "Value"=w1087) -> ()  [unwired: 2 in, 2 out]
                n674 = property on="Oxidizer" class="CmbBox"("Strings[]"=w1090, "Value"=w1087) -> ()  [unwired: 2 in, 2 out]
                n675 = property on="Initial Pressure" class="CmbBox"("Strings[]"=w1089, "Value"=w1087) -> ()  [unwired: 2 in, 2 out]
                n676 = property on="Equivalence Ratio" class="CmbBox"("Strings[]"=w1092, "Value"=w1087) -> ()  [unwired: 2 in, 2 out]
                n677 = property on="Diluent" class="CmbBox"("Strings[]"=w1093, "Value"=w1087) -> ()  [unwired: 2 in, 2 out]
                n678 = property on="Diluent Mole Fraction" class="CmbBox"("Strings[]"=w1094, "Value"=w1087) -> ()  [unwired: 2 in, 2 out]
                n679 = property on="Fuel" class="CmbBox"("DisabledEnum"=w1085) -> ()  [unwired: 2 in, 2 out]
                n680 = property on="Diluent Mole Fraction" class="CmbBox"("DisabledEnum"=w1085) -> ()  [unwired: 2 in, 2 out]
                n681 = property on="Initial Pressure" class="CmbBox"("DisabledEnum"=w1085) -> ()  [unwired: 2 in, 2 out]
                n682 = property on="Oxidizer" class="CmbBox"("DisabledEnum"=w1085) -> ()  [unwired: 2 in, 2 out]
                n683 = property on="Equivalence Ratio" class="CmbBox"("DisabledEnum"=w1085) -> ()  [unwired: 2 in, 2 out]
                n684 = property on="Diluent" class="CmbBox"("DisabledEnum"=w1085) -> ()  [unwired: 2 in, 2 out]
                n685 = local write "Test Status"("Test matrix loaded" ("Test Status")) -> ()
                "indices" <- w1088
              }
              frame Error {
              }
            }
          }
          event Timeout {
            n686 = event-data() -> ()  [unwired: 1 in, 1 out]
            n687 = local read "Set Mode"() -> (w1109:bool)
            n688 = case "Set to vent on timeout if vi is in Run Mode" shown="True" w1109 {
              tunnel: w1115 -> [w1118 w1125]
              tunnel: w1114 -> [w1117 w1124]
              tunnel: [w1118 w1123] -> w1113
              tunnel: [w1117 w1122] -> w1112
              tunnel: w1096 -> [_ w1119]
              frame False {
              }
              frame True {
                w1120 = T2."Tube Vent" ("State")
                n689 = Equal?(x=w1120, y=w1119) -> (x = y?=w1121:bool)
                n690 = case "and if it isn't already venting" shown="False" w1121 {
                  tunnel: w1125 -> [w1131 w1133]
                  tunnel: w1124 -> [w1130 w1134]
                  tunnel: [w1129 w1133] -> w1123
                  tunnel: [w1128 w1134] -> w1122
                  tunnel: w1120 -> [w1126 _]
                  frame False {
                    n691 = local read "valve\nrefs"() -> (w1132:refnum<vi>[])
                    n692 = control-ref of="Tube State"() -> (w1127:refnum<vi>)
                    n693 = call "Set Tube State.vi"("State"=w1126, "valve refs"=w1132, "error in"=w1130, "tube state ref"=w1127, "task in"=w1131) -> ("error out"=w1128:errorcluster, "task out"=w1129:refnum<k21>)  [unwired: 3 in]
                  }
                  frame True {
                  }
                }
              }
            }
            n694 = local read "Test Status"() -> (w1111:string)
            n695 = In Range and Coerce(upper limit=dbl[unit] 107300.0, x="Atmospheric Pressure", lower limit=dbl[unit] 95400.0) -> (In Range?=w1099:bool)  [unwired: 1 out]
            n696 = Equal?(x="Ready", y=w1111) -> (x = y?=w1097:bool)
            "tube ready?" <- w1097
            n697 = And(x=w1097, y=w1099) -> (x .and. y?=w1105:bool)
            n698 = Select(t=u32 0 ("Numeric Text.Text Colors:Text Color"), s=w1099, f=u32 16711680 ("Numeric Text.Text Colors:Text Color")) -> (s? t:f=w1098:u32)
            n699 = Select(t=T3."Enabled", s=w1105, f=T3."Disabled and Grayed Out" ("Disabled")) -> (s? t:f=w1102:T3)
            n700 = property on="Atmospheric Pressure" class="DigNum (strict)"("NumText.TextColor"=w1098) -> ()  [unwired: 2 in, 2 out]
            n701 = property on="Run Test" class="Bool"("DisabledEnum"=w1102) -> ()  [unwired: 2 in, 2 out]
            n702 = disable-structure "Disable individual controls in run mode" shown="Default" {
              frame Enabled {
                w1116 = T3."Disabled" ("Disabled")
                n703 = property on="Valve Diluent" class="Bool (strict)"("DisabledEnum"=w1116) -> ()  [unwired: 2 in, 2 out]
                n704 = property on="Valve Fuel" class="Bool (strict)"("DisabledEnum"=w1116) -> ()  [unwired: 2 in, 2 out]
                n705 = property on="Valve Mix Inlet" class="Bool (strict)"("DisabledEnum"=w1116) -> ()  [unwired: 2 in, 2 out]
                n706 = property on="Valve Mix Outlet" class="Bool (strict)"("DisabledEnum"=w1116) -> ()  [unwired: 2 in, 2 out]
                n707 = property on="Valve Oxidizer" class="Bool (strict)"("DisabledEnum"=w1116) -> ()  [unwired: 2 in, 2 out]
                n708 = property on="Valve Purge" class="Bool (strict)"("DisabledEnum"=w1116) -> ()  [unwired: 2 in, 2 out]
                n709 = property on="Valve Tube Inlet" class="Bool (strict)"("DisabledEnum"=w1116) -> ()  [unwired: 2 in, 2 out]
                n710 = property on="Valve Tube Outlet" class="Bool (strict)"("DisabledEnum"=w1116) -> ()  [unwired: 2 in, 2 out]
                n711 = property on="Valve Vacuum" class="Bool (strict)"("DisabledEnum"=w1116) -> ()  [unwired: 2 in, 2 out]
                n712 = property on="Mix Fan" class="Bool (strict)"("DisabledEnum"=w1116) -> ()  [unwired: 2 in, 2 out]
                n713 = property on="Tube State" class="Enum (strict)"("DisabledEnum"=w1116) -> ()  [unwired: 2 in, 2 out]
              }
            }
            n714 = local read "Stop"() -> (w1095:bool)
            n715 = property on="Stop all" class="Bool (strict)"("Val(Sgnl)"=w1095) -> ()  [unwired: 2 in, 2 out]
          }
          event "Initial Pressure", "Fuel", "Diluent", "Oxidizer", "Equivalence Ratio", "Diluent Mole Fraction": Value Change {
            # "since oxidizer is most of the mixture, let it soak up the vacuum error"
            n716 = event-data() -> ()  [unwired: 1 in, 1 out]
            n717 = local read "Test CSV"() -> (w1151:string[][])
            n718 = local read "indices"() -> (w1150:T1)
            n719 = call "Get Test Conditions.vi"("Fuel"="Fuel", "CSV Array"=w1151, "indices"=w1150, "Oxidizer"="Oxidizer", "Diluent"="Diluent", "Equivalence Ratio"="Equivalence Ratio", "Diluent Mole Fraction"="Diluent Mole Fraction", "Initial Pressure"="Initial Pressure") -> ("Test Found"=w1142:bool, "Fuel Cutoff Pressure"=w1148:dbl, "Test row"=w1143:string[], "Oxidizer Cutoff Pressure"=w1145:dbl, "f_a_st"=→"f_a_st":dbl, "Diluent Cutoff Pressure"=w1144:dbl)  [unwired: 2 in]
            n720 = local write "Test row"(w1143) -> ()
            n721 = node(w1144) -> (w1138:dbl[unit])
            n722 = node(w1148) -> (w1147:dbl[unit])
            n723 = node(w1145) -> (→"Oxidizer Cutoff (default)":dbl[unit])
            n724 = Select(t="Ready", s=w1142, f="No test found for these conditions") -> (s? t:f=w1139:string)
            n725 = Add(x="Vacuum Cutoff", y=w1138) -> (x+y=→"Diluent Cutoff (adjusted)" →"Diluent Cutoff (default)":dbl[unit])
            n726 = Add(x=w1147, y="Vacuum Cutoff") -> (x+y=→"Fuel Cutoff (adjusted)" →"Fuel Cutoff (default)":dbl[unit])
            n727 = local write "Test Status"(w1139) -> ()
          }
        }
      }
    }
    n728 = local read "Stop"() -> (w314:bool)
  }
  n729 = while {
    tunnel: w4 -> [w1164]
    tunnel: w3 -> [w1163]
    tunnel: [w1162] -> w2
    tunnel: [w1161] -> w1
    stop <- w1160 stop-if-true
    n730 = event shown="[1] \"Stop all\": Value Change" {
      selector: _ -> [_ _]
      dyn-events: _ -> [_ _]
      timeout: _ -> [_ _]
      tunnel: [_ "Stop all"] -> w1160
      tunnel: w1164 -> [w1165 w1182]
      tunnel: w1163 -> [w1166 w1181]
      tunnel: [w1166 w1168] -> w1161
      tunnel: [w1165 w1172] -> w1162
      event Timeout {
        n731 = event-data() -> ()  [unwired: 1 in, 3 out]
      }
      event "Stop all": Value Change {
        w1175 = "Shutting down" ("Test Status")
        w1167 = T2."Tube Vent" ("State")
        n732 = event-data() -> ()  [unwired: 1 in, 6 out]
        n733 = local read "valve\nrefs"() -> (w1171:refnum<vi>[])
        n734 = control-ref of="Tube State"() -> (w1170:refnum<vi>)
        n735 = local write "tube ready?"(FALSE ("tube ready?")) -> ()
        n736 = property on="Set Mode" class="Bool (strict)"("DisabledEnum"=T3."Disabled" ("Disabled")) -> ()  [unwired: 2 in, 2 out]
        n737 = property on="Run Test" class="Bool"("DisabledEnum"=T3."Enabled" ("Disabled")) -> ()  [unwired: 2 in, 2 out]
        n738 = call "Set Tube State.vi"("State"=w1167, "valve refs"=w1171, "error in"=w1182, "tube state ref"=w1170, "task in"=w1181) -> ("error out"=w1187:errorcluster, "task out"=w1180:refnum<k21>)  [unwired: 3 in]
        n739 = call "Wait Valve Actuate.vi"("error in"=w1187) -> ("error out"=w1185:errorcluster)
        n740 = disable-structure shown="Default" {
          disable-tunnel: w1185 -> [w1191]
          disable-tunnel: [w1191] -> w1184
          frame Enabled {
            n741 = Wait (ms)(milliseconds to wait=u32 5000) -> ()  [unwired: 1 out]
          }
        }
        n742 = To Upper Case(1:w1175) -> (0:w1174:string)
        n743 = call "Set Tube State.vi"("State"=T2."Manifold Vent", "valve refs"=w1171, "error in"=w1184, "tube state ref"=w1170, "task in"=w1180) -> ("error out"=w1186:errorcluster, "task out"=w1169:refnum<k21>)  [unwired: 3 in]
        n744 = local write "Test Status"(w1175) -> ()
        n745 = property on="tube ready?" class="Bool"("BoolText.Text"=w1174) -> ()  [unwired: 2 in, 2 out]
        n746 = property on="Set Mode" class="Bool (strict)"("BoolText.Text"=w1174) -> ()  [unwired: 2 in, 2 out]
        n747 = call "Wait Valve Actuate.vi"("error in"=w1186) -> ("error out"=w1183:errorcluster)
        n748 = disable-structure shown="Default" {
          disable-tunnel: w1183 -> [w1189]
          disable-tunnel: [w1189] -> w1173
          frame Enabled {
            n749 = Wait (ms)(milliseconds to wait=u32 5000) -> ()  [unwired: 1 out]
          }
        }
        n750 = call "Set Tube State.vi"("State"=w1167, "valve refs"=w1171, "error in"=w1173, "tube state ref"=w1170, "task in"=w1169) -> ("error out"=w1172:errorcluster, "task out"=w1168:refnum<k21>)  [unwired: 3 in]
      }
    }
    n751 = local write "Stop sensors"(w1160) -> ()
  }
  n752 = Merge Errors(w24, w17, w18, w19) -> (w23:errorcluster)
  n753 = disable-structure "Cleanup" shown="Default" {
    disable-tunnel: w29 -> [w1201]
    disable-tunnel: w27 -> [w1200]
    disable-tunnel: w25 -> [w1199]
    disable-tunnel: w23 -> [w1198]
    disable-tunnel: w7 -> [w1197]
    disable-tunnel: w6 -> [w1196]
    disable-tunnel: w5 -> [w1195]
    disable-tunnel: w1 -> [w1194]
    disable-tunnel: w2 -> [w1193]
    frame Enabled {
      n754 = disable-structure "Queues" shown="Default" {
        disable-tunnel: w1199 -> [w1218]
        disable-tunnel: w1198 -> [w1214]
        disable-tunnel: w1197 -> [w1215]
        frame Enabled {
          # "Pressure"
          # "Temperature"
          n755 = Flush Queue(queue=w1215, error in (no error)=w1214) -> (queue out=w1216:refnum<queue>, error out=w1217:errorcluster)  [unwired: 1 out]
          n756 = Flush Queue(queue=w1218, error in (no error)=w1214) -> (queue out=w1220:refnum<queue>, error out=w1219:errorcluster)  [unwired: 1 out]
          n757 = Release Queue(queue=w1216, error in (no error)=w1217) -> ()  [unwired: 1 in, 3 out]
          n758 = Release Queue(queue=w1220, error in (no error)=w1219) -> ()  [unwired: 1 in, 3 out]
        }
      }
      n759 = disable-structure "DAQ" shown="Default" {
        disable-tunnel: w1201 -> [w1213]
        disable-tunnel: w1200 -> [w1212]
        disable-tunnel: w1196 -> [w1207]
        disable-tunnel: w1195 -> [w1206]
        disable-tunnel: w1194 -> [w1204]
        disable-tunnel: w1193 -> [w1203]
        frame Enabled {
          # "DIO"
          # "Pressure"
          # "Temperature"
          n760 = call <vilib>:"DAQmx Stop Task.vi"("task/channels in"=w1207, "error in"=w1206) -> ("task out"=w1209:refnum<k21>, "error out"=w1208:errorcluster)  [unwired: 12 in]
          n761 = call <vilib>:"DAQmx Stop Task.vi"("task/channels in"=w1212, "error in"=w1213) -> ("task out"=w1211:refnum<k21>, "error out"=w1210:errorcluster)  [unwired: 12 in]
          n762 = call <vilib>:"DAQmx Stop Task.vi"("task/channels in"=w1204, "error in"=w1203) -> ("task out"=w1202:refnum<k21>, "error out"=w1205:errorcluster)  [unwired: 12 in]
          n763 = call <vilib>:"DAQmx Clear Task.vi"("task in"=w1209, "error in"=w1208) -> ()  [unwired: 13 in, 1 out]
          n764 = call <vilib>:"DAQmx Clear Task.vi"("task in"=w1211, "error in"=w1210) -> ()  [unwired: 13 in, 1 out]
          n765 = call <vilib>:"DAQmx Clear Task.vi"("task in"=w1202, "error in"=w1205) -> ()  [unwired: 13 in, 1 out]
        }
      }
    }
  }
